vi "WHD_VEten_0.1.3.WS_BIDIR_SAI_opt.vi"() -> ()   [LabVIEW 2015]
uses:
  <vilib>/NI_Real-Time Target Support.lvlib
  <vilib>/rvi/interface/nirviReadWriteControl/nirviReadWriteControl.xnode
  <vilib>/rvi/interface/nirviMethod/nirviMethod.xnode
  <vilib>/rvi/interface/nirviOpenFPGA/nirviOpenFPGA.xnode
  <vilib>/rvi/interface/nirviCloseFPGA/nirviCloseFPGA.xnode
  <vilib>/userdefined/High Color/nirio_resource_hc.ctl
  <vilib>/rvi/errors/niLvFpgaMergeErrorWithErrorCode.vi
  <vilib>/Utility/file.llb/Write Delimited Spreadsheet (string).vi
  <vilib>/RTwatchdog.llb/Watchdog expiration actions.ctl
  AURA_Wheel/Json2Labv.lvlib
  AURA_Wheel/AuraWheelAPI/AuraWheel.lvlib
  <vilib>/rvi/errors/niLvFpgaAdjustHostInterfaceError.vi
  NiFpgaLv.dll
  <vilib>/Utility/error.llb/Error Cluster From Error Code.vi
  <vilib>/LabVIEW Targets/FPGA/cRIO/shared/nicrio_ModuleControls/nicrio_cRIO-9234_DataRatesRing2.ctl
  <vilib>/FPGAPlugInAG/cRIO-9031/niLvFpga_Run_cRIO-9031.vi
  <vilib>/FPGAPlugInAG/cRIO-9031/niLvFpga_Reset_cRIO-9031.vi
  FPGA Bitfiles/W&RDArabia_FPGATarget_FPGA8a2wsBIdirec_yJvL9yuTbZw.lvbitx
  <vilib>/Utility/config.llb/NI_LVConfig.lvlib
  <vilib>/Utility/config.llb/Write Key (Double).vi
  <vilib>/platform/TimedLoop/XDataNode/XDataNode.xnode
  <vilib>/Platform/TimedLoop/XDataNode/nitl_modes.ctl
  <vilib>/Platform/TimedLoop/XDataNode/XDNodeRunTimeDep.lvlib
  <vilib>/Platform/TimedLoop/XDataNode/wakeup.ctl
  <vilib>/Platform/TimedLoop/XDataNode/timing_clust.ctl
  <vilib>/FPGAPlugInAG/cRIO-9031/niLvFpga_Open_cRIO-9031.vi
  <vilib>/FPGAPlugInAG/cRIO-9031/niLvFpga_ConfigureFifo_cRIO-9031.vi
  <vilib>/FPGAPlugInAG/cRIO-9031/niLvFpga_StartFifo_cRIO-9031.vi
  <vilib>/FPGAPlugInAG/cRIO-9031/niLvFpga_ReadFifo_cRIO-9031.vi
  <vilib>/FPGAPlugInAG/cRIO-9031/niLvFpga_StopFifo_cRIO-9031.vi
  <vilib>/FPGAPlugInAG/cRIO-9031/niLvFpga_Close_cRIO-9031.vi
panel:
  in  "Developer commad":string
  out "Save calibration":bool
  out "calibration log":path
  out "Pattern amplitude (g)":dbl=1.02
  out "Pattern frequency (Hz)":dbl=159.2
  out "Folder":path
  out "Report":string
  out "path calib":path
  out "AURA wheel test":bool
  out "LOG.txt":path
  out "Report_AURA":string
  out "RFID_Error":errorcluster
  out "error FPGA":errorcluster
  out "error AURA":errorcluster
  out "error manipulacion archivos":errorcluster
  out "Response headers":string
  out "Max RMS Ruedas":dbl[][](array[numeric])
  out "TAGs LR6":string[](array[string])
  out "TAGs HEX":string[](array[string])
  out "Parar":bool
  out "result":bool
  out "TAGs":string[](array[string])
  out "Temperatura (ºC)":dbl
  out "V (m/s)":dbl
  out "Digital?":bool=TRUE
  out "Watchdog config":T1={"reset system"=FALSE, "restart LabVIEW Runtime"=FALSE, "occurrence"=FALSE, "trigger protocol"=enum."active high", "trigger line"=enum."none", "disable watchdog on VI exit"=TRUE}
  out "Tiempo de adquisicion":dbl=10.0
  out "Adquirir":bool
  out "Nº Ruedas 1":i32
  out "NºRuedas 2":i32
  out "Disco Duro Disponible (bytes)":i64
  out "Buffer Overflow":bool
  out "Buffer Underflow":bool
  out "Archivo\nvalido?":bool
  out "Número de ejes detectados":i32
  out "Ejes_convoy":i32
  out "Tiempo de paso (s)":dbl
  out "created path":path
  out "Nombre de archivo":path[](array[path])
  out "LR6 IP address":string="192.168.106.94"
  out "Port LR6":u16=2001
  out "T fuera rango":bool
  out "Frecuencia de muestreo (Hz)":dbl=25600.0
  out "Escaneos de la FIFO por canal":u32=5000
  out "Tiempo extra al detector de paso (s)":dbl=1.0
  out "dt RMS":dbl=256.0
  out "Frecuencia de muestreo y módulo CRIO":T2=2 items=["51.200 kS/s (NI 9234)"=1, "25.600 kS/s (NI 9234)"=2, "17.067 kS/s (NI 9234)"=3, "12.800 kS/s (NI 9234)"=4, "10.240 kS/s (NI 9234)"=5, "8.533 kS/s (NI 9234)"=6, "7.314 kS/s (NI 9234)"=7, "6.400 kS/s (NI 9234)"=8, "5.689 kS/s (NI 9234)"=9, "5.120 kS/s (NI 9234)"=10, "4.654 kS/s (NI 9234)"=11, "4.267 kS/s (NI 9234)"=12, "3.938 kS/s (NI 9234)"=13, "3.657 kS/s (NI 9234)"=14, "3.413 kS/s (NI 9234)"=15, "3.200 kS/s (NI 9234)"=16, "3.012 kS/s (NI 9234)"=17, "2.845 kS/s (NI 9234)"=18, "2.695 kS/s (NI 9234)"=19, "2.560 kS/s (NI 9234)"=20, "2.438 kS/s (NI 9234)"=21, "2.328 kS/s (NI 9234)"=22, "2.226 kS/s (NI 9234)"=23, "2.133 kS/s (NI 9234)"=24, "2.048 kS/s (NI 9234)"=25, "1.969 kS/s (NI 9234)"=26, "1.896 kS/s (NI 9234)"=27, "1.829 kS/s (NI 9234)"=28, "1.765 kS/s (NI 9234)"=29, "1.707 kS/s (NI 9234)"=30, "1.652 kS/s (NI 9234)"=31]
  out "Puerto RFID":u16=2189
  out "IP RFID":string="192.168.106.99"
  out "Offset_rueda WS 2":fxp<+/-,24,-4>=0.004999998956918716 format="%.27g"
  out "Count(mSec)":u32=2
  out "RFID NEM on?":bool
  out "RFID LR6 on?":bool
  out "Canal cero WS1?":bool
  out "Canal cero WS2":bool
  out "Inicio pasada 2":timestamp
  in  "Calibration":bool
  out "Direccion 0?":bool
  out "Boton Adquirir?":bool
  out "RuedaDetectada2?":bool=TRUE
  out "RuedaDetectada1?":bool=TRUE
  out "Timeout ruedas":dbl
  out "Borrar archivos\nadquisicion con error":bool
  out "Able watchdog?":bool
  out "Reset watchdog?":bool
  out "Leer config RFID NEM":bool
  out "bytes to read":i32
  out "DeviceAddress":u8
  out "timeout ms (60000)":i32
  out "Max archivos":u32=2
  out "Bytes libre despues de borrar":u32=2
  out "Bytes min libre":u32=2
  out "Nº de acelerómetros":i32
  out "Nº inductivos":i32
  out "Offset_rueda WS 1":fxp<+/-,24,-4>=0.004999998956918716 format="%.27g"
  out "TAGs_AURAwheel":string[][](array[string])
  out "Plataformas?":bool
  out "Nº Ejes":i32[](array[numeric])
  out "Nº UTs":i32
  out "it-read-LR6":i32[](array[numeric])
  out "it-LR6":i32
  out "RFID_LR6_Error":errorcluster
  out "Series_flota":string[](array[string])
  out "Tabla_flota":string[][](array[string])
  out "Puntos medios de las ventanas":dbl[][](array[numeric])
  out "configuration file path":path=path "c:/Parametros.cfg"
  out "IP synchr":string
  out "data":cluster{"status":string}
  out "confRFID":path=path "c:/RFID/TAGS.csv"
  out "TAGS leidos":path=path "c:/RFID/TAGS.csv"
  out "Use Aura?":bool
  out "Parametros AuraWheel":string[](array[string])
  out "Parámetros acelerómetros":dbl[](array[numeric])
  out "Fin":bool
  out "Contador":i32=1
  out "Path LOG":path=path "c:/TEST"
  out "Fallo fotocelula":bool
  out "Path_Borrar":path=path "c:/Trenes"
  out "Longitud de la unidad":dbl
  out "Aviso no detección":string
  out "Time to Acquire Block (ms)":i32
  out "Distancia de acelerómetros":dbl[](array[numeric])
  out "Block Size":u32
  out "Distancias generales":dbl[](array[numeric])
  out "Reset del controlador":bool
  out "Parar la aplicación":bool
  out "date/time string":string
  out "Timeout ruedas":bool
  out "Tiempo":dbl
  out "Inicio pasada":timestamp
  out "Ultimo TEST":timestamp
  out "Fuente":bool=TRUE
  out "RFID_ID":refnum<k5>
  out "DC OK":string
  out "Aviso temperatura":string
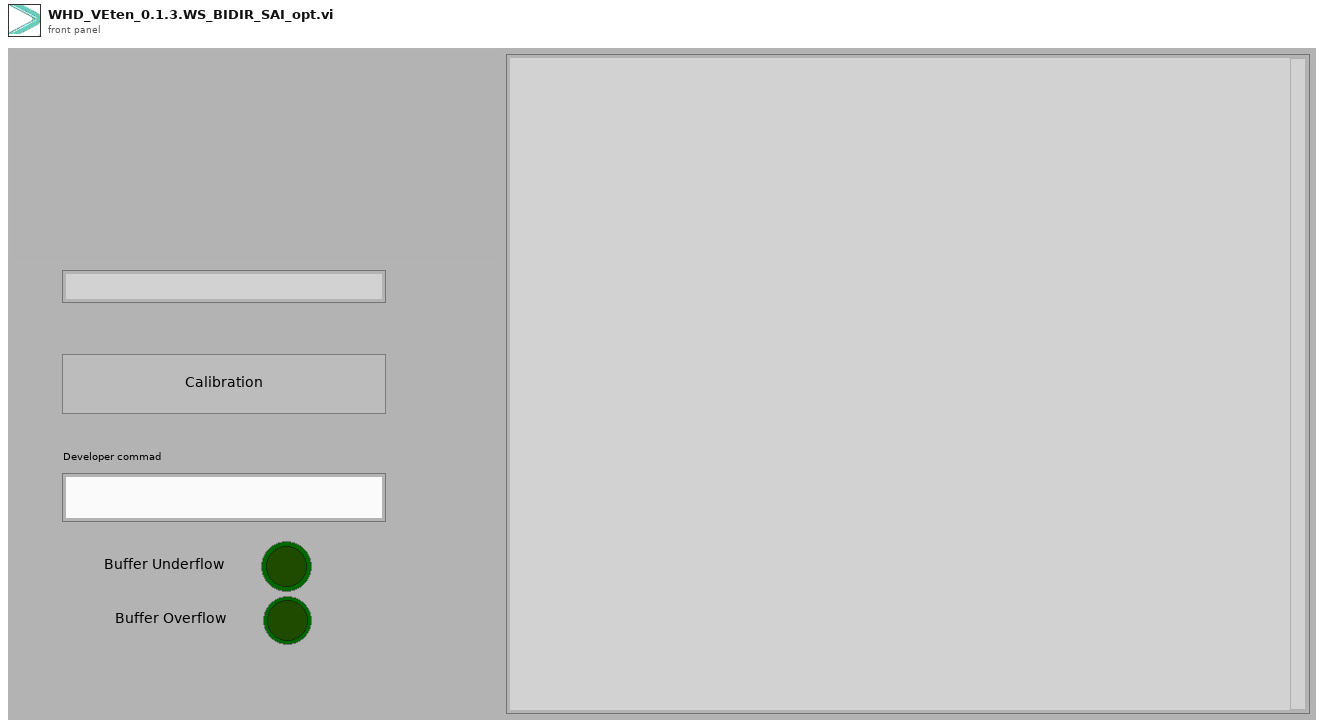
[diagram p1: front panel]
types:
  T1 = typedef "Watchdog expiration actions.ctl" = cluster{"reset system":bool, "restart LabVIEW Runtime":bool, "occurrence":bool, "trigger protocol":enum16{"active high", "active low", "open collector"}, "trigger line":enum16{"none", "line 0", "line 1", "line 2", "line 3", "line 4", "line 5", "line 6", "line 7", "SMB line 0"}, "disable watchdog on VI exit":bool}
  T2 = typedef "nicrio_cRIO-9234_DataRatesRing2.ctl" = u8
  T3 = typedef "nirio_resource_hc.ctl" = tag
  T4 = enum16{"Standard", "Buffered", "CRLF", "Immediate"}
  T5 = enum16{"open", "replace", "create", "open or create", "replace or create", "replace or create with confirmation"}
  T6 = enum16{"big-endian, network order", "native, host order", "little-endian"}
  T7 = typedef "XDNodeRunTimeDep.lvlib/timing_clust.ctl" = cluster{"Expected End [f-1]":u64, "Actual End [f-1]":u64, "Finished Late? [f-1]":bool, "Expected End [i-1]":u64, "Actual End [i-1]":u64, "Finished Late? [i-1]":bool, "Expected Start [i]":u64, "Actual Start [i]":u64, "Expected Start [f]":u64, "Actual Start [f]":u64, "Source Name":string, "Structure Name":string, "Period":i64, "Deadline":i64, "Offset":i64, "Start":i64, "Priority":i32, "Timeout":i32, "Mode":T8, "Wakeup Reason":T9, "Error":errorcluster, "Source Type":string, "Secondary Source Type":string, "Global End Time":u64, "Global Start Time":u64, "Frame Duration":u64, "Iteration Duration":u64, "Assigned CPU":i32, "I/O Scan Engine Mode":u32}
  T8 = typedef "XDNodeRunTimeDep.lvlib/nitl_modes.ctl" = enum32{"No Change", "Process missed periods, maintain original phase", "Discard missed periods, maintain original phase", "Process missed periods, ignore original phase", "Discard missed periods, ignore original phase"}
  T9 = typedef "XDNodeRunTimeDep.lvlib/wakeup.ctl" = enum32{"Normal", "Aborted", "Asynchronous wakeup", "Timing source error", "Timed loop error", "Timeout"}
  T10 = cluster{"error IO":errorcluster, bool[], u32[], string[], dbl[]}
  T11 = cluster{"error out":errorcluster, dbl[], "TAGs":string[], "Direccion 0?":bool}
  T12 = cluster{"g_ts":dbl, "p_sp":dbl, "p_tp":dbl, "p_tg":cluster{"tg_n":dbl, "tg_t":string}[], "p_ax":cluster{"ax_n":dbl, "ax_sp":dbl, "ax_wh":cluster{"wh_p":dbl, "wh_a1":dbl, "wh_a2":dbl, "wh_a3":dbl, "wh_a4":dbl}[]}[]}
  T13 = cluster{"Frecuencia de muestreo y módulo CRIO":T2, "Count(mSec)":u32, "Frecuencia de muestreo (Hz)":dbl, "Escaneos de la FIFO por canal":u32, "Nº inductivos":i32, "Nº de acelerómetros":i32}
  T14 = typedef "NI_LVConfig.lvlib/Config Data RefNum.ctl" = refnum<k1>
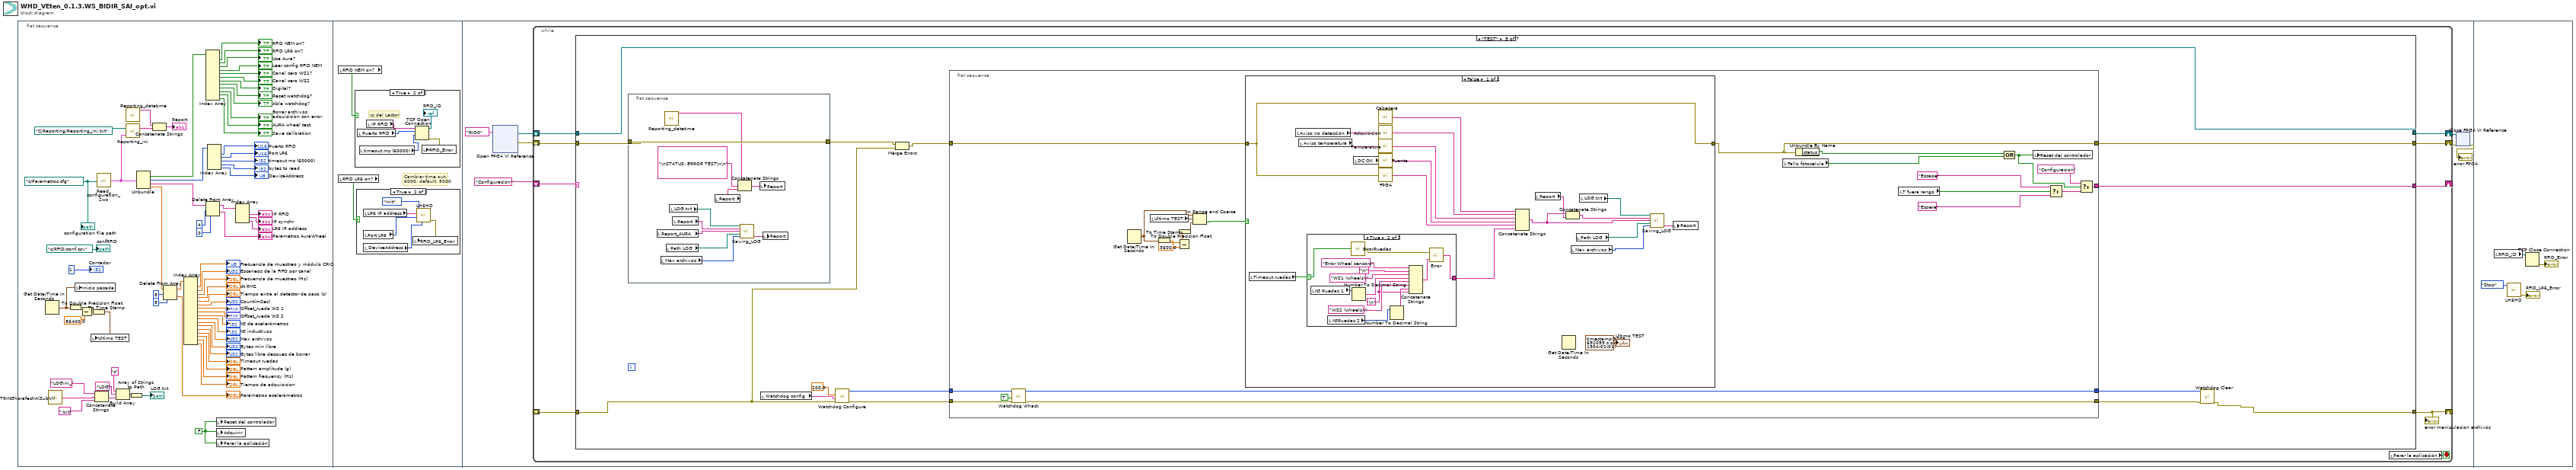
[diagram p0: block diagram]
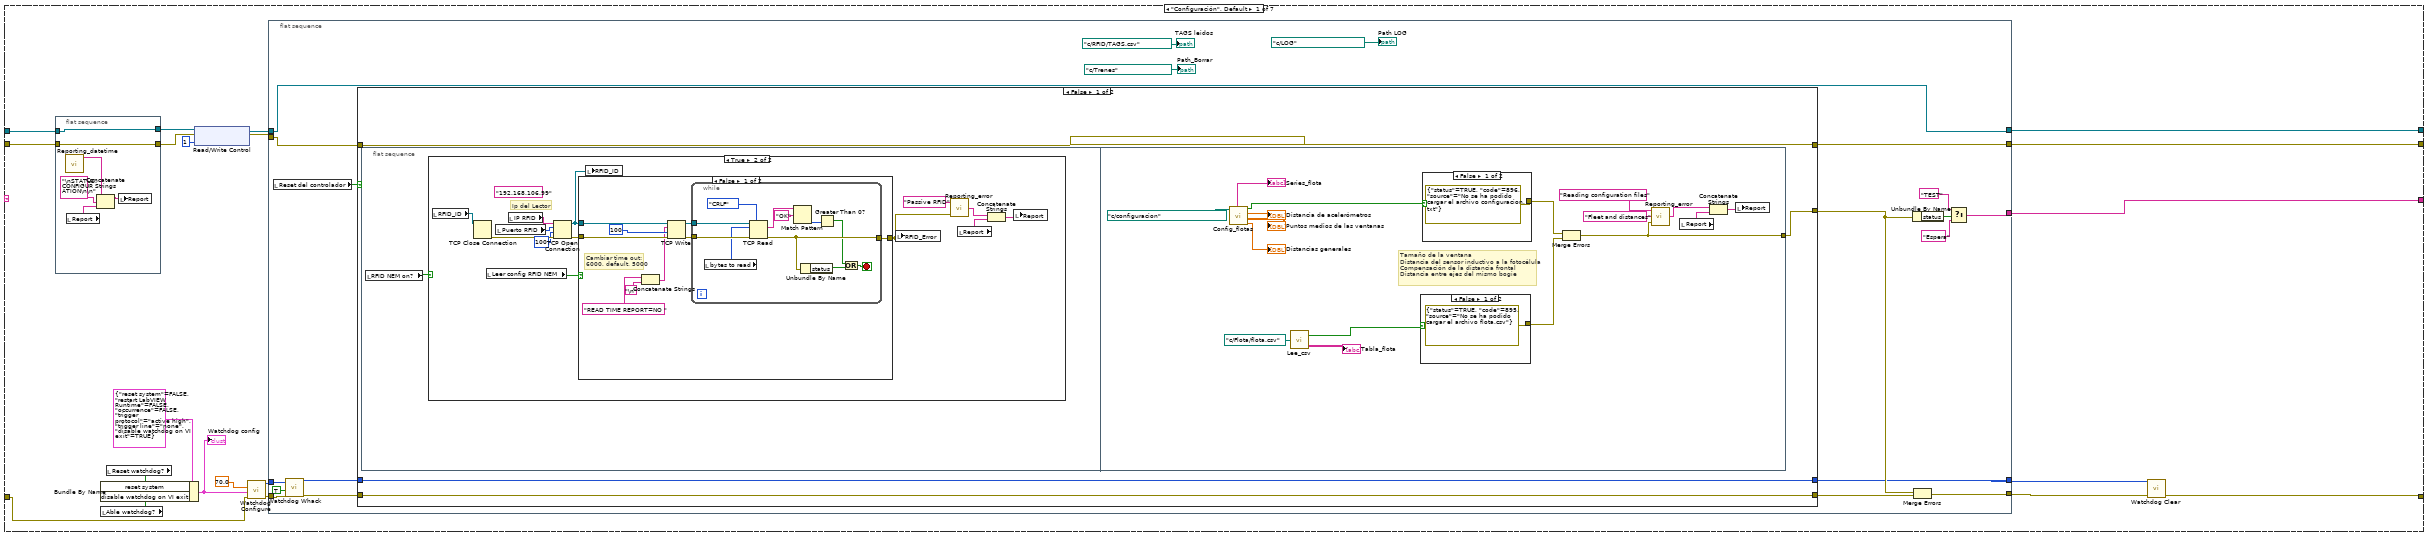
[diagram p4: hidden frame]
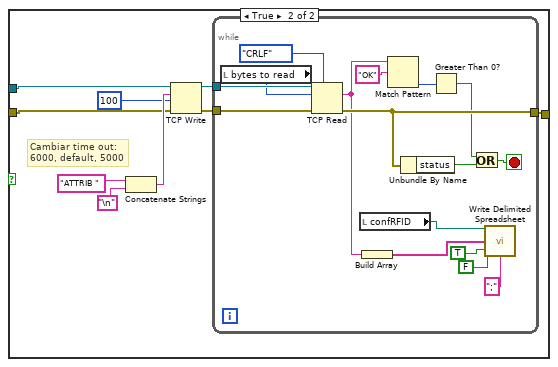
[diagram p6: hidden frame]
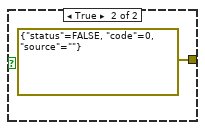
[diagram p7: hidden frame]
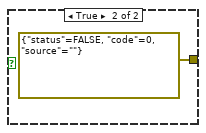
[diagram p8: hidden frame]
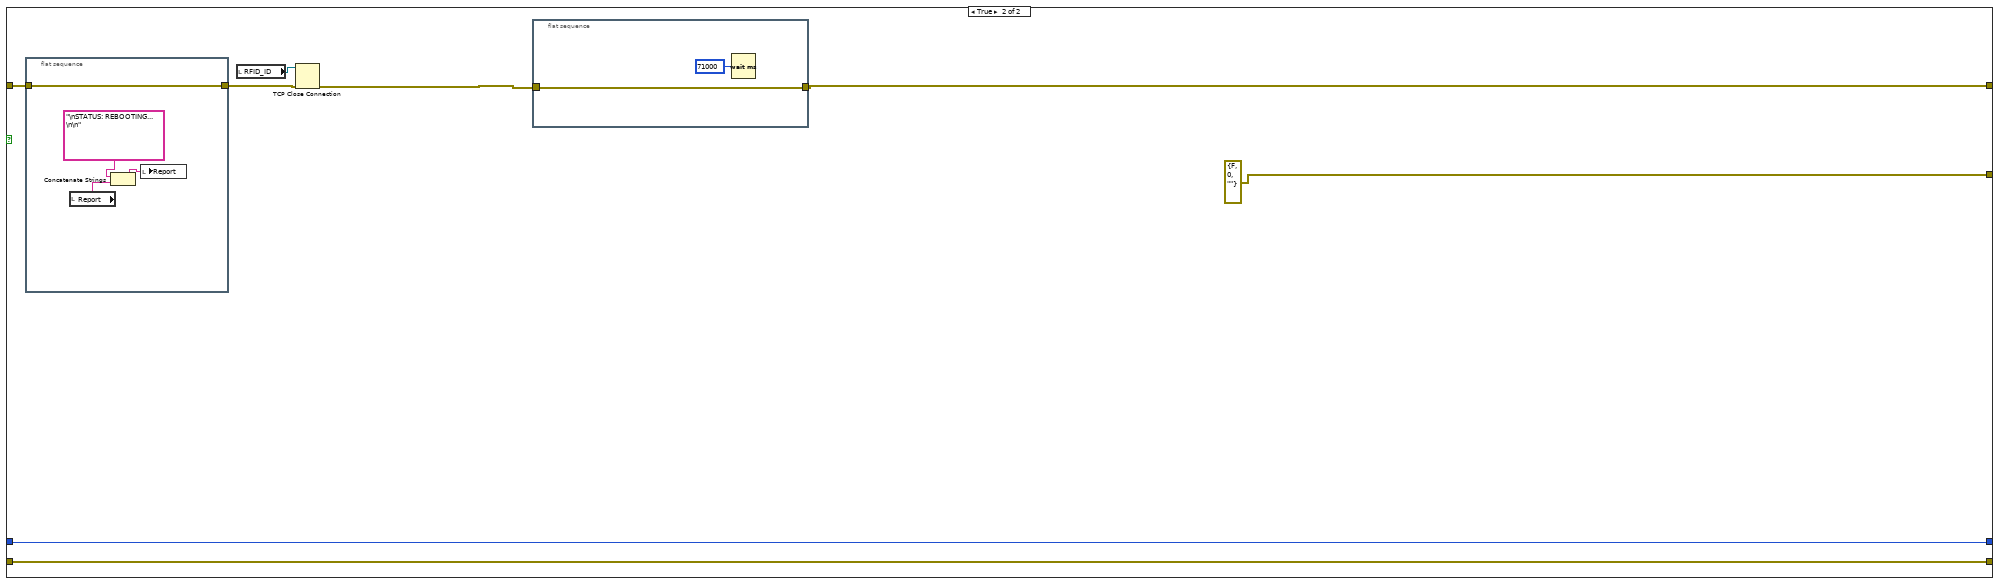
[diagram p9: hidden frame]
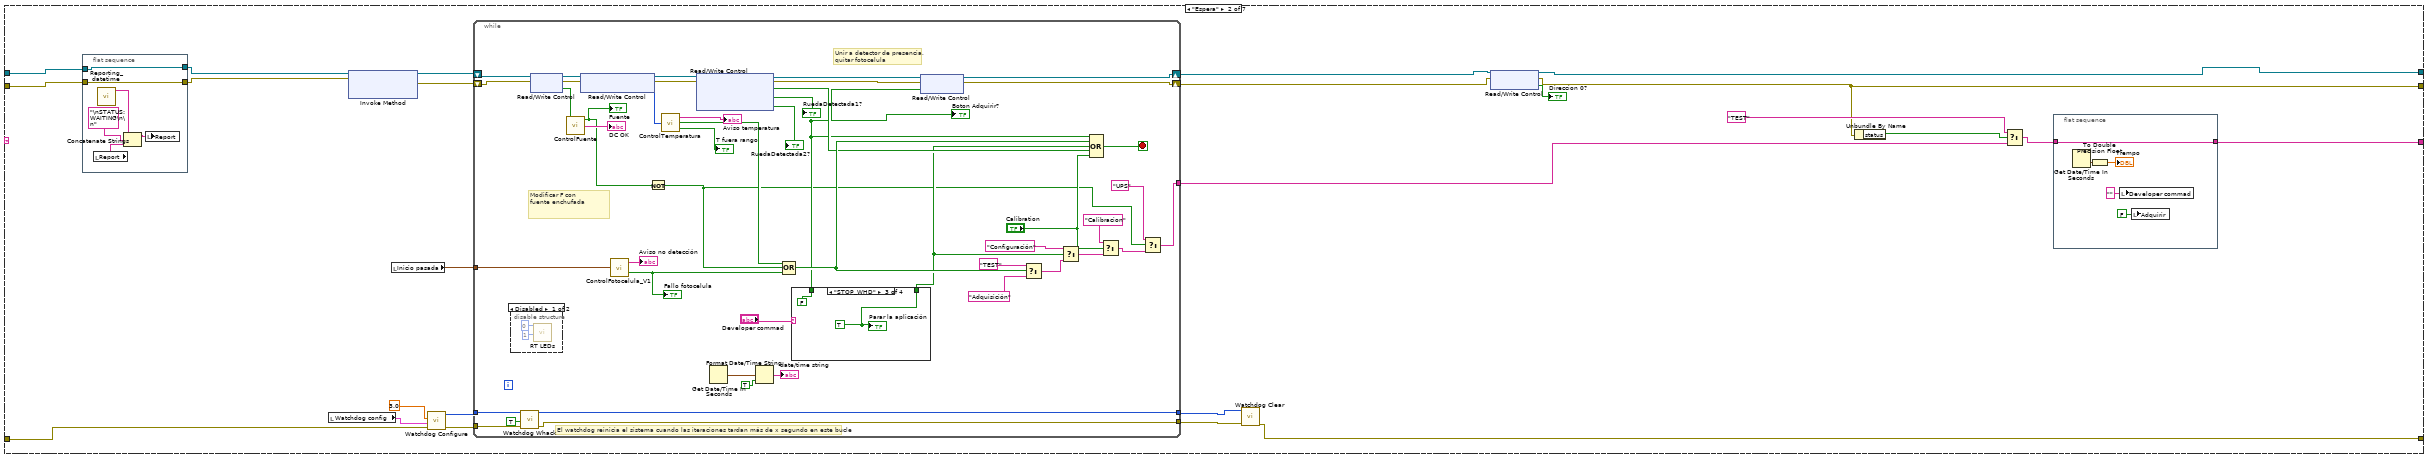
[diagram p10: hidden frame]
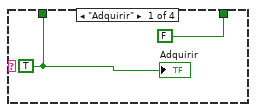
[diagram p11: hidden frame]
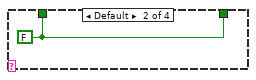
[diagram p12: hidden frame]
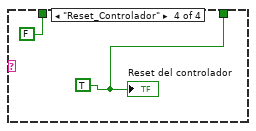
[diagram p13: hidden frame]
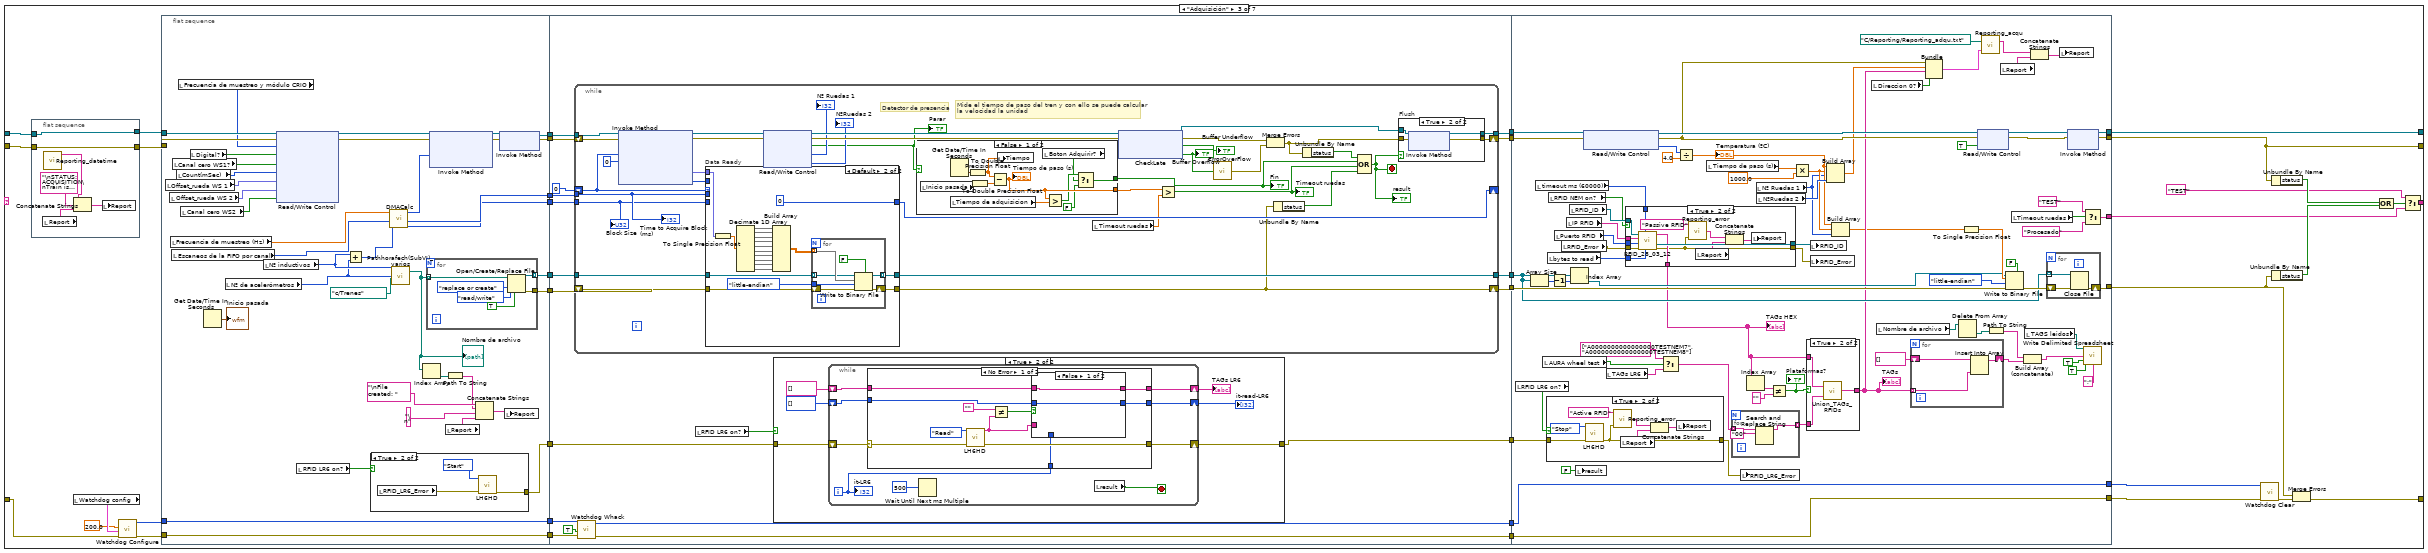
[diagram p15: hidden frame]
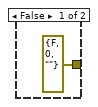
[diagram p16: hidden frame]
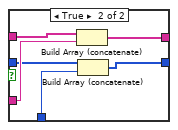
[diagram p18: hidden frame]
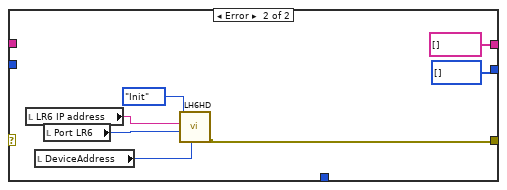
[diagram p19: hidden frame]
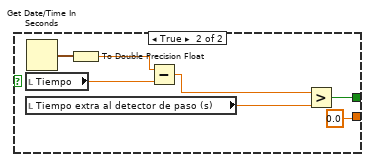
[diagram p20: hidden frame]
diagram:
  n1 = flat-sequence {
    frame #0 {
      w1 = FALSE ("Reset del controlador")
      w63 = path "c:/Parametros.cfg" ("configuration file path")
      n2 = Get Date/Time In Seconds() -> (seconds since 1Jan1904=w68:timestamp)
      n3 = call "STRINGhorafechA(SubVI).vi"() -> ("STRINGhora_fecha"=w12:string)
      n4 = To Double Precision Float(number=w68) -> (double precision float=w70:dbl)
      n5 = local write "Inicio pasada"(w68) -> ()
      n6 = Subtract(x=w70, y=86400.0) -> (x-y=w69:dbl)
      n7 = To Time Stamp(1:w69) -> (0:w67:timestamp)
      n8 = local write "Ultimo TEST"(w67) -> ()
      n9 = Concatenate Strings("LOGini_" ("string"), w12, ".txt" ("string")) -> (w14:string)
      n10 = call "Read_configuration_2ws.vi"("configuration file path"=w63) -> ("output cluster"=w18:T10)
      n11 = Build Array("c", "LOG" ("element"), w14) -> (w11:string[])
      n12 = call "Reporting_ini.vi"("Configuration cluster"=w18, "address repoting"=path "C:/Reporting/Reporting_ini.txt" ("file (use dialog)")) -> ("Reporting"=w17:string)  [unwired: 1 in]
      n13 = call "Reporting_datetime.vi"() -> ("String"=w15:string)  [unwired: 11 in]
      n14 = Array of Strings to Path(0:w11) -> (2:→"LOG.txt":path)  [unwired: 1 out]
      n15 = Unbundle(w18) -> (w66:bool[], w65:u32[], w58:string[], w62:dbl[])  [unwired: 1 out]
      n16 = Concatenate Strings(w15, w17) -> (→"Report":string)
      n17 = Delete From Array(array=w62, length=8, index=8) -> (deleted portion=→"Parámetros acelerómetros":dbl[], array with subset deleted=w61:dbl[])
      n18 = Index Array(array=w61) -> (element #1=→"Frecuencia de muestreo y módulo CRIO":dbl, element #2=→"Escaneos de la FIFO por canal":dbl, element #3=→"Frecuencia de muestreo (Hz)":dbl, element #4=→"dt RMS":dbl, element #5=→"Tiempo extra al detector de paso (s)":dbl, element #6=→"Count(mSec)":dbl, element #7=→"Offset_rueda WS 1":dbl, element #8=→"Offset_rueda WS 2":dbl, element #9=→"Nº de acelerómetros":dbl, element #10=→"Nº inductivos":dbl, element #11=→"Max archivos":dbl, element #12=→"Bytes min libre":dbl, element #13=→"Bytes libre despues de borrar":dbl, element #14=→"Timeout ruedas":dbl, element #15=→"Pattern amplitude (g)":dbl, element #16=→"Pattern frequency (Hz)":dbl, element #17=→"Tiempo de adquisicion":dbl)  [unwired: 17 in]
      n19 = Index Array(array=w66) -> (element #1=→"RFID NEM on?":bool, element #2=→"RFID LR6 on?":bool, element #3=→"Use Aura?":bool, element #4=→"Leer config RFID NEM":bool, element #5=→"Canal cero WS1?":bool, element #6=→"Canal cero WS2":bool, element #7=→"Digital?":bool, element #8=→"Reset watchdog?":bool, element #9=→"Able watchdog?":bool, element #10=→"Borrar archivos\nadquisicion con error":bool, element #11=→"AURA wheel test":bool, element #12=→"Save calibration":bool)  [unwired: 12 in]
      n20 = Delete From Array(array=w58, length=4, index=0) -> (deleted portion=→"Parametros AuraWheel":string[], array with subset deleted=w57:string[])
      n21 = Index Array(array=w65) -> (element #1=→"Puerto RFID":u32, element #2=→"Port LR6":u32, element #3=→"timeout ms (60000)":u32, element #4=→"bytes to read":u32, element #5=→"DeviceAddress":u32)  [unwired: 5 in]
      n22 = local write "Reset del controlador"(w1) -> ()
      n23 = local write "Adquirir"(w1) -> ()
      n24 = local write "Parar la aplicación"(w1) -> ()
      n25 = Index Array(array=w57) -> (element #1=→"IP RFID":string, element #2=→"IP synchr":string, element #3=→"LR6 IP address":string)  [unwired: 3 in]
      "Contador" <- 1
      "confRFID" <- path "c:/RFID/conf.csv" ("file path (use dialog)")
      "configuration file path" <- w63
    }
    frame #1 {
      # "Cambiar time out:\n6000, default, 5000"
      n26 = local read "RFID NEM on?"() -> (w73:bool)
      n27 = local read "RFID LR6 on?"() -> (w72:bool)
      n28 = case shown="True" w73 {
        frame False {
        }
        frame True {
          # "Ip del Lector"
          n29 = local read "Puerto RFID"() -> (w81:u16)
          n30 = local read "timeout ms (60000)"() -> (w79:i32)
          n31 = local read "IP RFID"() -> (w82:string)
          n32 = TCP Open Connection(address=w82, remote port or service name=w81, timeout ms (60000)=w79) -> (connection ID=→"RFID_ID":refnum<k5>, error out=w80:errorcluster)  [unwired: 1 in, 1 out]
          n33 = local write "RFID_Error"(w80) -> ()
        }
      }
      n34 = case shown="True" w72 {
        frame False {
        }
        frame True {
          n35 = local read "LR6 IP address"() -> (w74:string)
          n36 = local read "Port LR6"() -> (w75:u16)
          n37 = local read "DeviceAddress"() -> (w76:u8)
          n38 = call "LH6HD.vi"("DeviceAddress"=w76, "Reader Port"=w75, "IP Address"=w74, "Action"=enum16{"Init", "Start", "Read", "Stop", "Exit"}."Init") -> ("error out"=w78:errorcluster)  [unwired: 6 in, 1 out]
          n39 = local write "RFID_LR6_Error"(w78) -> ()
        }
      }
    }
    frame #2 {
      n40 = xnode "Open FPGA VI Reference"("resource name"=T3 "RIO0") -> ("FPGA VI Reference Out"=w90:refnum<k20>, "error out"=w89:errorcluster)  [unwired: 1 in]
      n41 = while {
        shift-right: [w91] -> _
        shift-left: "Configuración" -> [w99]
        shift-right: [w93] -> w86
        shift-left: w90 -> [w98]
        shift-right: [w92] -> w85
        shift-left: w89 -> [w97]
        shift-right: [w96] -> _
        shift-left: _ -> [w95]
        stop <- w94 stop-if-true
        n42 = case shown="\"TEST\"" w99 {
          tunnel: [w109 w262 w354 w711 w959 "Espera" "Espera" ("t")] -> w91
          tunnel: [w119 w250 w368 w700 w958 w1038 w1229] -> w93
          tunnel: [w120 w249 w369 w698 w957 w1037 w1228] -> w92
          tunnel: w98 -> [w103 w248 w340 w701 w958 w1043 w1232]
          tunnel: w97 -> [w102 w247 w339 w699 w950 w1042 w1231]
          tunnel: [w116 w256 w366 w696 w949 _ _] -> w96
          tunnel: w95 -> [w108 w261 w350 w710 w946 _ _]
          frame "Configuración", Default {
            n43 = flat-sequence {
              tunnel: w103 -> [w126]
              tunnel: w102 -> [w125]
              tunnel: [w126] -> w101
              tunnel: [w125] -> w100
              frame #0 {
                n44 = call "Reporting_datetime.vi"() -> ("String"=w121:string)  [unwired: 11 in]
                n45 = local read "Report"() -> (w122:string)
                n46 = Concatenate Strings(w121, "\nSTATUS: CONFIGURATION\n\n", w122) -> (w124:string)
                n47 = local write "Report"(w124) -> ()
              }
            }
            n48 = local read "Able watchdog?"() -> (w113:bool)
            n49 = local read "Reset watchdog?"() -> (w114:bool)
            n50 = Bundle By Name(cluster=T1 {"reset system"=FALSE, "restart LabVIEW Runtime"=FALSE, "occurrence"=FALSE, "trigger protocol"=enum."active high", "trigger line"=enum."none", "disable watchdog on VI exit"=TRUE} ("expiration actions"), "reset system"=w114, "disable watchdog on VI exit"=w113) -> (w107:T1)
            "Watchdog config" <- w107
            n51 = xnode "Read/Write Control"("FPGA VI Reference In"=w101, "error in"=w100, "Cycles to Filter"=u16 1) -> ("FPGA VI Reference Out"=w112:refnum<k20>, "error out"=w111:errorcluster)
            n52 = call <vilib>:"Watchdog Configure.vi"("error in (no error)"=w108, "expiration actions"=w107, "timeout (1 sec)"=70.0) -> ("error out"=w104:errorcluster, "watchdogID"=w105:u64)  [unwired: 1 in, 2 out]
            n53 = flat-sequence {
              tunnel: [w137] -> w120
              tunnel: [w145] -> w109
              tunnel: w112 -> [w138]
              tunnel: [w138] -> w119
              tunnel: [w140] -> w117
              tunnel: w111 -> [w135]
              tunnel: [w132] -> w118
              tunnel: w105 -> [w128]
              tunnel: w104 -> [w127]
              frame #0 {
                n54 = local read "Reset del controlador"() -> (w134:bool)
                n55 = call <vilib>:"Watchdog Whack.vi"("error in (no error)"=w127, "reset watchdog after expire? (F)"=TRUE, "watchdogID in"=w128) -> ("error out"=w130:errorcluster, "watchdogID out"=w131:u64)  [unwired: 2 in, 1 out]
                n56 = case shown="False" w134 {
                  tunnel: w135 -> [w150 w233]
                  tunnel: [w150 w236] -> w137
                  tunnel: [w147 errorcluster {"status"=FALSE, "code"=0, "source"=""} ("error IO")] -> w136
                  tunnel: [w149 w235] -> w132
                  tunnel: w131 -> [w149 w235]
                  tunnel: w130 -> [w148 w234]
                  tunnel: [w148 w234] -> w129
                  frame False {
                    n57 = flat-sequence {
                      tunnel: [w210] -> w147
                      frame #0 {
                        n58 = local read "RFID NEM on?"() -> (w151:bool)
                        n59 = case shown="True" w151 {
                          frame False {
                          }
                          frame True {
                            (unwired) "192.168.106.99" ("address")
                            # "Ip del Lector"
                            n60 = local read "RFID_ID"() -> (w163:refnum<k5>)
                            n61 = TCP Close Connection(connection ID=w163) -> (error out=w164:errorcluster)  [unwired: 2 in, 1 out]
                            n62 = local read "Leer config RFID NEM"() -> (w157:bool)
                            n63 = local read "Puerto RFID"() -> (w161:u16)
                            n64 = local read "IP RFID"() -> (w160:string)
                            n65 = TCP Open Connection(address=w160, remote port or service name=w161, timeout ms (60000)=100, error in (no error)=w164) -> (connection ID=w162:refnum<k5>, error out=w158:errorcluster)  [unwired: 1 out]
                            n66 = case shown="False" w157 {
                              tunnel: w162 -> [w173 w187]
                              tunnel: [w171 w185] -> w156
                              tunnel: w158 -> [w168 w186]
                              frame False {
                                # "Cambiar time out:\n6000, default, 5000"
                                n67 = Concatenate Strings("READ TIME REPORT=NO " ("data in"), "\n") -> (w165:string)
                                n68 = TCP Write(connection ID=w173, data in=w165, error in (no error)=w168, 9:100 ("timeout ms (25000)")) -> (connection ID out=w169:refnum<k5>, error out=w170:errorcluster)  [unwired: 1 out]
                                n69 = while {
                                tunnel: w170 -> [w183]
                                tunnel: w169 -> [w182]
                                tunnel: [w181] -> w171
                                stop <- w178 stop-if-true
                                n70 = local read "bytes to read"() -> (w174:i32)
                                n71 = TCP Read(connection ID=w182, bytes to read=w174, error in (no error)=w183, 7:T4."CRLF" ("mode (standard)")) -> (data out=w176:string, error out=w181:errorcluster)  [unwired: 1 in, 1 out]
                                n72 = Match Pattern(string=w176, regular expression="OK") -> (offset past match=w179:i32)  [unwired: 4 out]
                                n73 = Unbundle By Name(w181) -> ("status"=w177:bool)
                                n74 = Greater Than 0?(x=w179) -> (x > 0?=w175:bool)
                                n75 = Or(x=w175, y=w177) -> (x .or. y?=w178:bool)
                                }
                              }
                              frame True {
                                # "Cambiar time out:\n6000, default, 5000"
                                n76 = Concatenate Strings("ATTRIB " ("data in"), "\n") -> (w193:string)
                                n77 = TCP Write(connection ID=w187, data in=w193, error in (no error)=w186, 9:100 ("timeout ms (25000)")) -> (connection ID out=w190:refnum<k5>, error out=w189:errorcluster)  [unwired: 1 out]
                                n78 = while {
                                tunnel: w189 -> [w208]
                                tunnel: w190 -> [w207]
                                tunnel: [w206] -> w185
                                stop <- w203 stop-if-true
                                n79 = local read "bytes to read"() -> (w194:i32)
                                n80 = TCP Read(connection ID=w207, bytes to read=w194, error in (no error)=w208, 7:T4."CRLF" ("mode (standard)")) -> (data out=w197:string, error out=w206:errorcluster)  [unwired: 1 in, 1 out]
                                n81 = local read "confRFID"() -> (w196:path)
                                n82 = Build Array(w197) -> (w195:string[])
                                n83 = Match Pattern(string=w197, regular expression="OK") -> (offset past match=w204:i32)  [unwired: 4 out]
                                n84 = Unbundle By Name(w206) -> ("status"=w202:bool)
                                n85 = Greater Than 0?(x=w204) -> (x > 0?=w201:bool)
                                n86 = Or(x=w201, y=w202) -> (x .or. y?=w203:bool)
                                n87 = call-poly <vilib>:"Write Delimited Spreadsheet.vi"("file path (dialog if empty)"=w196, "1D data"=w195, "append to file? (new file:F)"=FALSE ("transpose? (no:F)"), "transpose? (no:F)"=TRUE ("append to file? (new file:F)"), "delimiter (\\t)"=";" ("delimiter (\\t)")) -> ()  [unwired: 9 in, 2 out]
                                }
                              }
                            }
                            n88 = local write "RFID_ID"(w162) -> ()
                            n89 = local write "RFID_Error"(w156) -> ()
                            n90 = call "Reporting_error.vi"("error out 2"=w156, "Concept"="Passive RFID") -> ("Reporting"=w153:string)  [unwired: 1 in]
                            n91 = local read "Report"() -> (w154:string)
                            n92 = Concatenate Strings(w153, w154) -> (w152:string)
                            n93 = local write "Report"(w152) -> ()
                          }
                        }
                      }
                      frame #1 {
                        # "Tamaño de la ventana\nDistancia del sensor inductivo a la fotocélula\nCompensación de la distancia frontal\nDistancia entre ejes del mismo bogie"
                        n94 = call "Config_flotas.vi"("file path (dialog if empty)"=path "c:/configuracion") -> ("Distancias generales"=→"Distancias generales":dbl[], "Puntos medios de las ventanas"=→"Puntos medios de las ventanas":dbl[][], "Distancia de acelerómetros"=→"Distancia de acelerómetros":dbl[], "Distacias y medidas de dispositivos"=w223:bool, "Series_flota"=→"Series_flota":string[])  [unwired: 3 in]
                        n95 = call "Lee_csv.vi"("Path"=path "c:/Flota/flota.csv") -> ("Tabla_flota"=→"Tabla_flota":string[][], "Lectura_OK?"=w220:bool)
                        n96 = case shown="False" w220 {
                          tunnel: [errorcluster {"status"=TRUE, "code"=895, "source"="No se ha podido cargar el archivo flota.csv"} ("error out") errorcluster {"status"=FALSE, "code"=0, "source"=""} ("error out")] -> w224
                          frame False {
                          }
                          frame True {
                          }
                        }
                        n97 = case shown="False" w223 {
                          tunnel: [errorcluster {"status"=TRUE, "code"=896, "source"="No se ha podido cargar el archivo configuracion.txt"} ("error out") errorcluster {"status"=FALSE, "code"=0, "source"=""} ("error out")] -> w225
                          frame False {
                          }
                          frame True {
                          }
                        }
                        n98 = Merge Errors(w225, w224) -> (w210:errorcluster)
                        n99 = call "Reporting_error.vi"("error out 2"=w210, "Concept explanation"="Fleet and distances", "Concept"="Reading configuration files") -> ("Reporting"=w212:string)
                        n100 = local read "Report"() -> (w211:string)
                        n101 = Concatenate Strings(w212, w211) -> (w213:string)
                        n102 = local write "Report"(w213) -> ()
                      }
                    }
                  }
                  frame True {
                    n103 = flat-sequence {
                      tunnel: w233 -> [w242]
                      tunnel: [w242] -> w232
                      frame #0 {
                        n104 = local read "Report"() -> (w241:string)
                        n105 = Concatenate Strings("\nSTATUS: REBOOTING...\n\n", w241) -> (w239:string)
                        n106 = local write "Report"(w239) -> ()
                      }
                    }
                    n107 = local read "RFID_ID"() -> (w238:refnum<k5>)
                    n108 = TCP Close Connection(connection ID=w238, error in (no error)=w232) -> (error out=w231:errorcluster)  [unwired: 2 out]
                    n109 = flat-sequence {
                      tunnel: [w244] -> w236
                      tunnel: w231 -> [w244]
                      frame #0 {
                        n110 = Wait (ms)(milliseconds to wait=u32 71000) -> ()  [unwired: 1 out]
                      }
                    }
                  }
                }
                n111 = Unbundle By Name(w136) -> ("status"=w146:bool)
                n112 = Merge Errors(w136, w129) -> (w140:errorcluster)
                n113 = Select(t="TEST", s=w146, f="Espera") -> (s? t:f=w145:string)
                "Path_Borrar" <- path "c:/Trenes" ("file path (use dialog)")
                "Path LOG" <- path "c:/LOG" ("file path (use dialog)")
                "TAGS leidos" <- path "c:/RFID/TAGS.csv" ("file path (use dialog)")
              }
            }
            n114 = call <vilib>:"Watchdog Clear.vi"("error in (no error)"=w117, "watchdogID in"=w118) -> ("error out"=w116:errorcluster)  [unwired: 5 in]
          }
          frame "Espera" {
            n115 = flat-sequence {
              tunnel: w248 -> [w275]
              tunnel: w247 -> [w274]
              tunnel: [w275] -> w246
              tunnel: [w274] -> w245
              frame #0 {
                n116 = local read "Report"() -> (w271:string)
                n117 = call "Reporting_datetime.vi"() -> ("String"=w270:string)  [unwired: 11 in]
                n118 = Concatenate Strings(w270, "\nSTATUS: WAITING\n\n", w271) -> (w273:string)
                n119 = local write "Report"(w273) -> ()
              }
            }
            n120 = local read "Watchdog config"() -> (w255:T1)
            n121 = xnode "Invoke Method"("FPGA VI Reference In"=w246, "error in"=w245) -> ("FPGA VI Reference Out"=w265:refnum<k20>, "error out"=w264:errorcluster)  [unwired: 1 in]
            n122 = local read "Inicio pasada"() -> (w269:timestamp)
            n123 = call <vilib>:"Watchdog Configure.vi"("error in (no error)"=w261, "expiration actions"=w255, "timeout (1 sec)"=3.0) -> ("error out"=w260:errorcluster, "watchdogID"=w259:u64)  [unwired: 1 in, 2 out]
            n124 = while {
              tunnel: [w282] -> w268
              shift-right: [w299] -> w251
              shift-left: w265 -> [w307]
              shift-right: [w298] -> w252
              shift-left: w264 -> [w306]
              tunnel: w269 -> [w310]
              tunnel: w260 -> [w296]
              tunnel: w259 -> [w297]
              tunnel: [w295] -> w258
              tunnel: [w294] -> w257
              stop <- w289 stop-if-true
              # "Modificar F con\nfuente enchufada"
              # "Unir a detector de presencia,\nquitar fotocelula"
              # "El watchdog reinicia el sistema cuando las iteraciones tardan más de x segundo en este bucle"
              n125 = disable-structure shown="Disabled" {
                frame Disabled {
                  n126 = call <vilib>:"RT LEDs.vi"("State"=1, "LED Num"=0) -> ()  [unwired: 1 in, 5 out]
                }
                frame Enabled {
                }
              }
              n127 = call <vilib>:"Watchdog Whack.vi"("error in (no error)"=w296, "reset watchdog after expire? (F)"=TRUE, "watchdogID in"=w297) -> ("error out"=w294:errorcluster, "watchdogID out"=w295:u64)  [unwired: 2 in, 1 out]
              n128 = xnode "Read/Write Control"("FPGA VI Reference In"=w307, "error in"=w306) -> ("FPGA VI Reference Out"=w319:refnum<k20>, "error out"=w318:errorcluster, "DC OK"=w323:bool)
              n129 = call "ControlFuente.vi"("DC OK 3"=w323) -> ("DC OK 2"=w283:bool, "DC OK"=→"DC OK":string)  [unwired: 1 out]
              "Fuente" <- w283
              n130 = xnode "Read/Write Control"("FPGA VI Reference In"=w319, "error in"=w318) -> ("FPGA VI Reference Out"=w314:refnum<k20>, "error out"=w313:errorcluster, "Chassis Temperature"=w321:i16)
              n131 = call "ControlFotocelula_V1.vi"("Tiempo de entrada a espera"=w310) -> ("Aviso no detección"=→"Aviso no detección":string, "Boolean"=w311:bool)
              "Fallo fotocelula" <- w311
              n132 = Not(x=w283) -> (.not. x?=w281:bool)
              n133 = call "ControlTemperatura.vi"("Chassis Temperature"=w321) -> ("Aviso temperatura"=→"Aviso temperatura":string, "Boolean"=w315:bool, "T fuera rango"=→"T fuera rango":bool)
              n134 = xnode "Read/Write Control"("FPGA VI Reference In"=w314, "error in"=w313) -> ("FPGA VI Reference Out"=w309:refnum<k20>, "error out"=w308:errorcluster, "Detector de presencia"=w302:bool, "RuedaDetectada1?"=→"RuedaDetectada1?":bool, "RuedaDetectada2?"=→"RuedaDetectada2?":bool)
              n135 = Get Date/Time In Seconds() -> (seconds since 1Jan1904=w304:timestamp)
              n136 = Format Date/Time String(seconds (now)=w304, UTC format=TRUE) -> (date/time string=→"date/time string":string)  [unwired: 1 in]
              n137 = Compound Arithmetic op=OR(w315, w281, w311) -> (w312:bool)
              n138 = case shown="\"STOP_WHD\"" "Developer commad" {
                tunnel: [w329 w330 FALSE ("Adquirir") FALSE ("Adquirir")] -> w288
                tunnel: [FALSE ("Adquirir") w330 w331 w333] -> w287
                frame "Adquirir" {
                  w329 = TRUE ("Adquirir")
                  "Adquirir" <- w329
                }
                frame Default {
                  w330 = FALSE ("Adquirir")
                }
                frame "STOP_WHD" {
                  w331 = TRUE ("Adquirir")
                  "Parar la aplicación" <- w331
                }
                frame "Reset_Controlador" {
                  w333 = TRUE ("Adquirir")
                  "Reset del controlador" <- w333
                }
              }
              "Boton Adquirir?" <- w288
              n139 = xnode "Read/Write Control"("FPGA VI Reference In"=w309, "error in"=w308, "Fotocélula"=w288) -> ("FPGA VI Reference Out"=w299:refnum<k20>, "error out"=w298:errorcluster)
              n140 = Select(t="TEST", s=w312, f="Adquisición") -> (s? t:f=w324:string)
              n141 = Select(t="Configuración", s=w287, f=w324) -> (s? t:f=w292:string)
              n142 = Compound Arithmetic op=OR(w288, w312, w287, w302, "Calibration") -> (w289:bool)
              n143 = Select(t="Calibracion", s="Calibration", f=w292) -> (s? t:f=w285:string)
              n144 = Select(t="UPS", s=w281, f=w285) -> (s? t:f=w282:string)
            }
            n145 = call <vilib>:"Watchdog Clear.vi"("error in (no error)"=w257, "watchdogID in"=w258) -> ("error out"=w256:errorcluster)  [unwired: 5 in]
            n146 = xnode "Read/Write Control"("FPGA VI Reference In"=w251, "error in"=w252) -> ("FPGA VI Reference Out"=w250:refnum<k20>, "error out"=w249:errorcluster, "Direccion 0?"=→"Direccion 0?":bool)
            n147 = Unbundle By Name(w249) -> ("status"=w267:bool)
            n148 = Select(t="TEST", s=w267, f=w268) -> (s? t:f=w263:string)
            n149 = flat-sequence {
              tunnel: [w279] -> w262
              tunnel: w263 -> [w279]
              frame #0 {
                n150 = Get Date/Time In Seconds() -> (seconds since 1Jan1904=w280:timestamp)
                n151 = To Double Precision Float(number=w280) -> (double precision float=→"Tiempo":dbl)
                n152 = local write "Developer commad"("" ("Developer commad")) -> ()
                n153 = local write "Adquirir"(FALSE ("Adquirir")) -> ()
              }
            }
          }
          frame "Adquisición" {
            n154 = flat-sequence {
              tunnel: w340 -> [w380]
              tunnel: w339 -> [w379]
              tunnel: [w380] -> w338
              tunnel: [w379] -> w337
              frame #0 {
                n155 = local read "Report"() -> (w376:string)
                n156 = call "Reporting_datetime.vi"() -> ("String"=w375:string)  [unwired: 11 in]
                n157 = Concatenate Strings(w375, "\nSTATUS: ACQUISITION\nTrain is passing\n\n", w376) -> (w378:string)
                n158 = local write "Report"(w378) -> ()
              }
            }
            n159 = local read "Watchdog config"() -> (w351:T1)
            n160 = call <vilib>:"Watchdog Configure.vi"("error in (no error)"=w350, "expiration actions"=w351, "timeout (1 sec)"=200.0) -> ("error out"=w348:errorcluster, "watchdogID"=w349:u64)  [unwired: 1 in, 2 out]
            n161 = flat-sequence {
              tunnel: w337 -> [w414]
              tunnel: w338 -> [w415]
              tunnel: [w413] -> w365
              tunnel: [w412] -> w364
              tunnel: [w411] -> w363
              tunnel: [w410] -> w362
              tunnel: [w409] -> w361
              tunnel: [w408] -> w360
              tunnel: [w398] -> w353
              tunnel: w349 -> [w397]
              tunnel: w348 -> [w396]
              tunnel: [w397] -> w347
              tunnel: [w396] -> w346
              tunnel: [w430] -> w374
              tunnel: [w447] -> w373
              tunnel: [w446] -> w372
              tunnel: [w445] -> w371
              tunnel: [w438] -> w370
              tunnel: w365 -> [w444]
              tunnel: w364 -> [w443]
              tunnel: w363 -> [w442]
              tunnel: w362 -> [w441]
              tunnel: w361 -> [w440]
              tunnel: w360 -> [w439]
              tunnel: w353 -> [w436]
              tunnel: [w435] -> w352
              tunnel: w347 -> [w434]
              tunnel: w346 -> [w433]
              tunnel: [w431] -> w345
              tunnel: w374 -> [w611]
              tunnel: w373 -> [w606]
              tunnel: w372 -> [w605]
              tunnel: w371 -> [w625]
              tunnel: [w652] -> w357
              tunnel: w370 -> [w654]
              tunnel: [w641] -> w367
              tunnel: [w642] -> w369
              tunnel: [w643] -> w368
              tunnel: w352 -> [w620]
              tunnel: w345 -> [w612]
              tunnel: [w612] -> w343
              tunnel: [w611] -> w342
              frame #0 {
                n162 = local read "Offset_rueda WS 1"() -> (w391:fxp<+/-,24,-4>)
                n163 = local read "Offset_rueda WS 2"() -> (w392:fxp<+/-,24,-4>)
                n164 = local read "Frecuencia de muestreo (Hz)"() -> (w406:dbl)
                n165 = local read "Escaneos de la FIFO por canal"() -> (w395:u32)
                n166 = local read "Canal cero WS1?"() -> (w400:bool)
                n167 = local read "Count(mSec)"() -> (w399:u32)
                n168 = local read "Frecuencia de muestreo y módulo CRIO"() -> (w402:T2)
                n169 = local read "Canal cero WS2"() -> (w390:bool)
                n170 = local read "Digital?"() -> (w401:bool)
                n171 = Get Date/Time In Seconds() -> (seconds since 1Jan1904=→"Inicio pasada":timestamp)
                n172 = local read "Nº de acelerómetros"() -> (w388:i32)
                n173 = local read "Nº inductivos"() -> (w389:i32)
                n174 = xnode "Read/Write Control"("FPGA VI Reference In"=w415, "error in"=w414, "Data Rate"=w402, "Digital?"=w401, "Canal cero WS1?"=w400, "Count(mSec)"=w399, "Offset_WS1"=w391, "Offset_WS2"=w392, "Canal cero WS2?"=w390) -> ("FPGA VI Reference Out"=w405:refnum<k20>, "error out"=w404:errorcluster)
                n175 = local read "RFID LR6 on?"() -> (w393:bool)
                n176 = Add(x=w389, y=w388) -> (x+y=w394:i32)
                n177 = case shown="True" w393 {
                  tunnel: [errorcluster {"status"=FALSE, "code"=0, "source"=""} ("error out") w420] -> w398
                  frame False {
                  }
                  frame True {
                    n178 = local read "RFID_LR6_Error"() -> (w421:errorcluster)
                    n179 = call "LH6HD.vi"("error in (no error)"=w421, "Action"=enum16{"Init", "Start", "Read", "Stop", "Exit"}."Start") -> ("error out"=w420:errorcluster)  [unwired: 8 in, 1 out]
                  }
                }
                n180 = call "DMACalc.vi"("Number of Channels"=w394, "Number of Samples"=w395, "Rate (Hz)"=w406) -> ("Block Size"=w410:u32, "Time to Acquire Block (ms)"=w411:i32, "Host Buffer Size"=w416:u32)  [unwired: 6 in]
                n181 = call "Pathhorafech(SubVI)_varios.vi"("Folder path"=path "c:/Trenes", "Nº de acelerómetros"=w388, "Nº inductivos"=w389) -> ("Acel_Paths"=w384:path[])  [unwired: 1 in, 1 out]
                "Nombre de archivo" <- w384
                n182 = Index Array(array=w384) -> (element=w383:path)  [unwired: 1 in]
                n183 = for {
                  tunnel: w384 -> [w425] mode=indexing
                  tunnel: [w424] -> w409 mode=indexing
                  tunnel: [w423] -> w408
                  n184 = Open/Create/Replace File(file path (use dialog)=w425, operation (0:open)=T5."replace or create", access (0:read/write)=enum16{"read/write", "read-only", "write-only"}."read/write", disable buffering (F)=TRUE) -> (refnum out=w424:refnum<file>, error out=w423:errorcluster)  [unwired: 1 in, 2 out]
                }
                n185 = xnode "Invoke Method"("FPGA VI Reference In"=w405, "error in"=w404, "Requested Depth"=w416) -> ("FPGA VI Reference Out"=w418:refnum<k20>, "error out"=w417:errorcluster)  [unwired: 1 out]
                n186 = local read "Report"() -> (w387:string)
                n187 = Path To String(path=w383) -> (string=w381:string)
                n188 = Concatenate Strings("\nFile created: ", w381, "\n", w387) -> (w386:string)
                n189 = xnode "Invoke Method"("FPGA VI Reference In"=w418, "error in"=w417) -> ("FPGA VI Reference Out"=w413:refnum<k20>, "error out"=w412:errorcluster)
                n190 = local write "Report"(w386) -> ()
              }
              frame #1 {
                n191 = while "Data Acquisition" {
                  tunnel: w444 -> [w498]
                  shift-right: [w522] -> _
                  shift-left: u32 0 ("t") -> [w518]
                  tunnel: w442 -> [w523]
                  tunnel: w441 -> [w521]
                  shift-right: [w524] -> w446
                  shift-left: w443 -> [w515]
                  tunnel: [w519] -> w447
                  tunnel: w440 -> [w502]
                  tunnel: [w503] -> w445
                  shift-right: [w501] -> w438
                  shift-left: w439 -> [w511]
                  stop <- w520 stop-if-true
                  # "Detector de presencia"
                  # "Mide el tiempo de paso del tren y con ello se puede calcular\nla velocidad la unidad"
                  n192 = xnode "Invoke Method"("FPGA VI Reference In"=w498, "error in"=w515, "Number of Elements"=w518, "Timeout (ms)"=0) -> ("FPGA VI Reference Out"=w495:refnum<k20>, "error out"=w500:errorcluster, "Data"=w514:fxp<+/-,24,4>[], "Elements Remaining"=w516:u32)
                  n193 = case "Data Ready" shown="Default" w518 {
                    tunnel: w523 -> [w546 _]
                    tunnel: [w545 u32 0 ("t")] -> w522
                    tunnel: w521 -> [w547 _]
                    tunnel: w516 -> [w544 _]
                    tunnel: w514 -> [_ w569]
                    tunnel: w511 -> [w543 w568]
                    tunnel: [w543 w570] -> w501
                    tunnel: w502 -> [w542 w567]
                    tunnel: [w542 w566] -> w503
                    frame 0 {
                      # "En este caso se compara los elementos que quedan\nen la FIFO del controlador con el tamaño dell bloque\nque aparece en el panel frontal. Si el número de \nelementos en la FIFO es mayor o igual que el tamaño\n del bloque se pasa al siguiente caso y se guardan \nlos datos en un archivo. El reloj que aparece es una\nespera para no consumir recursos."
                      n194 = Greater Or Equal?(x=w544, y=w547) -> (x >= y?=w548:bool)
                      n195 = case shown="False" w548 {
                        tunnel: [u32 0 ("Block Size") w552] -> w545
                        tunnel: [w551 0 ("t")] -> w549
                        tunnel: w546 -> [w551 _]
                        tunnel: w547 -> [_ w552]
                        frame False {
                        }
                        frame True {
                        }
                      }
                      n196 = call "WaitMinTimeBetweenCall.vi"("Minimum ms between calls"=w549) -> ()  [unwired: 2 in]
                    }
                    frame Default {
                      n197 = To Single Precision Float(number=w569) -> (single precision float=w556:sgl[])
                      n198 = Decimate 1D Array(w556) -> (w562:sgl[], w565:sgl[], w564:sgl[], w563:sgl[], w561:sgl[], w560:sgl[], w559:sgl[], w558:sgl[], w557:sgl[], w554:sgl[])
                      n199 = Build Array(w562, w565, w564, w563, w561, w560, w559, w558, w557, w554) -> (w555:sgl[][])
                      n200 = for {
                        tunnel: T6."little-endian" ("byte order (0:big-endian, network order)") -> [w579]
                        shift-right: [w573] -> w570
                        shift-left: w568 -> [w574]
                        tunnel: w555 -> [w577] mode=indexing
                        tunnel: w567 -> [w576] mode=indexing
                        tunnel: [w575] -> w566 mode=indexing
                        n201 = Write to Binary File(file (use dialog)=w576, data=w577, error in=w574, 5:FALSE ("prepend array or string size? (T)"), 9:w579) -> (refnum out=w575:refnum<file>, error out=w573:errorcluster)  [unwired: 2 out]
                      }
                    }
                  }
                  n202 = xnode "Read/Write Control"("FPGA VI Reference In"=w495, "error in"=w500) -> ("FPGA VI Reference Out"=w513:refnum<k20>, "error out"=w512:errorcluster, "Parar"=w491:bool, "Nº Ruedas 1"=→"Nº Ruedas 1":i32, "NºRuedas 2"=→"NºRuedas 2":i32)
                  "Parar" <- w491
                  n203 = case shown="False" w491 {
                    tunnel: [w529 w537] -> w492
                    tunnel: [w530 0.0] -> w506
                    frame False {
                      n204 = local read "Inicio pasada"() -> (w533:timestamp)
                      n205 = Get Date/Time In Seconds() -> (seconds since 1Jan1904=w532:timestamp)
                      n206 = local read "Tiempo de adquisicion"() -> (w525:dbl)
                      n207 = To Double Precision Float(number=w532) -> (double precision float=w531:dbl)
                      n208 = To Double Precision Float(number=w533) -> (double precision float=w534:dbl)
                      n209 = Subtract(x=w531, y=w534) -> (x-y=w530:dbl)
                      "Tiempo de paso (s)" <- w530
                      n210 = local write "Tiempo"(w531) -> ()
                      n211 = local read "Boton Adquirir?"() -> (w526:bool)
                      n212 = Greater?(x=w530, y=w525) -> (0:w528:bool)
                      n213 = Select(t=w528, s=w526, f=FALSE) -> (s? t:f=w529:bool)
                    }
                    frame True {
                      n214 = local read "Tiempo"() -> (w541:dbl)
                      n215 = local read "Tiempo extra al detector de paso (s)"() -> (w536:dbl)
                      n216 = Get Date/Time In Seconds() -> (seconds since 1Jan1904=w538:timestamp)
                      n217 = To Double Precision Float(number=w538) -> (double precision float=w539:dbl)
                      n218 = Subtract(x=w539, y=w541) -> (x-y=w540:dbl)
                      n219 = Greater?(x=w540, y=w536) -> (0:w537:bool)
                    }
                  }
                  "Fin" <- w492
                  n220 = local read "Timeout ruedas"() -> (w490:dbl)
                  n221 = xnode ("CheckLate")("FPGA VI Reference In"=w513, "error in"=w512) -> ("FPGA VI Reference Out"=w497:refnum<k20>, "error out"=w508:errorcluster, "Buffer Underflow"=→"Buffer Underflow":bool, "Buffer Overflow"=w499:bool)
                  "Buffer Overflow" <- w499
                  n222 = Greater?(x=w506, y=w490) -> (0:w504:bool)
                  "Timeout ruedas" <- w504
                  n223 = call "ErrorOverFlow.vi"("Buffer Overflow"=w499) -> ("error out"=w507:errorcluster)
                  n224 = Merge Errors(w508, w507) -> (w496:errorcluster)
                  n225 = Unbundle By Name(w501) -> ("status"=w505:bool)
                  n226 = Unbundle By Name(w496) -> ("status"=w510:bool)
                  n227 = Compound Arithmetic op=OR(w510, w492, w504, w505) -> (w520:bool)
                  "result" <- w520
                  n228 = case "Flush" shown="True" w520 {
                    tunnel: [w580 w585] -> w524
                    tunnel: [w581 w584] -> w519
                    tunnel: w497 -> [w581 w583]
                    tunnel: w496 -> [w580 w582]
                    frame False {
                    }
                    frame True {
                      n229 = xnode "Invoke Method"("FPGA VI Reference In"=w583, "error in"=w582) -> ("FPGA VI Reference Out"=w584:refnum<k20>, "error out"=w585:errorcluster)
                    }
                  }
                  "Block Size" <- w521
                  "Time to Acquire Block (ms)" <- w523
                }
                n230 = call <vilib>:"Watchdog Whack.vi"("error in (no error)"=w433, "reset watchdog after expire? (F)"=TRUE, "watchdogID in"=w434) -> ("error out"=w430:errorcluster, "watchdogID out"=w431:u64)  [unwired: 2 in, 1 out]
                n231 = local read "RFID LR6 on?"() -> (w429:bool)
                n232 = case shown="True" w429 {
                  tunnel: w436 -> [w448 w454]
                  tunnel: [w448 w453] -> w435
                  frame False {
                  }
                  frame True {
                    n233 = while {
                      shift-right: [w461] -> w453
                      shift-left: w454 -> [w462]
                      shift-right: [w460] -> w451
                      shift-left: string[] [] -> [w459]
                      shift-right: [w455] -> w449
                      shift-left: i32[] [] -> [w456]
                      i -> [w457]
                      stop <- w458 stop-if-true
                      n234 = case shown="No Error" w462 {
                        selector: w462 -> [w473 _]
                        tunnel: [w472 w488] -> w461
                        tunnel: [w468 string[] []] -> w460
                        tunnel: w459 -> [w467 _]
                        tunnel: w457 -> [w466 _]
                        tunnel: w456 -> [w465 _]
                        tunnel: [w464 i32[] []] -> w455
                        frame No Error {
                          n235 = call "LH6HD.vi"("error in (no error)"=w473, "Action"=enum16{"Init", "Start", "Read", "Stop", "Exit"}."Read") -> ("error out"=w472:errorcluster, "Tag"=w469:string)  [unwired: 8 in]
                          n236 = Not Equal?(x="", y=w469) -> (x != y?=w470:bool)
                          n237 = case shown="False" w470 {
                            tunnel: w469 -> [_ w482]
                            tunnel: [w476 w481] -> w468
                            tunnel: w467 -> [w476 w480]
                            tunnel: w466 -> [_ w477]
                            tunnel: w465 -> [w475 w479]
                            tunnel: [w475 w478] -> w464
                            frame False {
                            }
                            frame True {
                              n238 = Build Array (concatenate)(w480, w482) -> (w481:string[])
                              n239 = Build Array (concatenate)(w479, w477) -> (w478:i32[])
                            }
                          }
                        }
                        frame Error {
                          n240 = local read "LR6 IP address"() -> (w485:string)
                          n241 = local read "DeviceAddress"() -> (w483:u8)
                          n242 = local read "Port LR6"() -> (w486:u16)
                          n243 = call "LH6HD.vi"("DeviceAddress"=w483, "Reader Port"=w486, "IP Address"=w485, "Action"=enum16{"Init", "Start", "Read", "Stop", "Exit"}."Init") -> ("error out"=w488:errorcluster)  [unwired: 6 in, 1 out]
                        }
                      }
                      n244 = Wait Until Next ms Multiple(millisecond multiple=u32 500) -> ()  [unwired: 1 out]
                      n245 = local read "result"() -> (w458:bool)
                      "it-LR6" <- w457
                    }
                    "TAGs LR6" <- w451
                    "it-read-LR6" <- w449
                  }
                }
              }
              frame #2 {
                n246 = local read "RFID LR6 on?"() -> (w607:bool)
                n247 = Array Size(array=w625) -> (size(s)=w623:i32)
                n248 = local read "timeout ms (60000)"() -> (w610:i32)
                n249 = local read "AURA wheel test"() -> (w587:bool)
                n250 = case shown="True" w607 {
                  tunnel: w620 -> [w660 w666]
                  tunnel: [w660 w661] -> w619
                  frame False {
                  }
                  frame True {
                    n251 = call "LH6HD.vi"("error in (no error)"=w666, "Action"=enum16{"Init", "Start", "Read", "Stop", "Exit"}."Stop") -> ("error out"=w661:errorcluster)  [unwired: 8 in, 1 out]
                    n252 = call "Reporting_error.vi"("error out 2"=w661, "Concept"="Active RFID") -> ("Reporting"=w663:string)  [unwired: 1 in]
                    n253 = local read "Report"() -> (w664:string)
                    n254 = Concatenate Strings(w663, w664) -> (w662:string)
                    n255 = local write "Report"(w662) -> ()
                  }
                }
                n256 = local read "bytes to read"() -> (w609:i32)
                n257 = local read "RFID NEM on?"() -> (w608:bool)
                n258 = Decrement(x=w623) -> (x-1=w624:i32)
                n259 = local read "Puerto RFID"() -> (w640:u16)
                n260 = local read "RFID_Error"() -> (w650:errorcluster)
                n261 = local read "IP RFID"() -> (w622:string)
                n262 = local read "RFID_ID"() -> (w649:refnum<k5>)
                n263 = Index Array(array=w625, index=w624) -> (element=w633:refnum<file>)
                n264 = local write "result"(FALSE ("result")) -> ()
                n265 = xnode "Read/Write Control"("FPGA VI Reference In"=w606, "error in"=w605) -> ("FPGA VI Reference Out"=w651:refnum<k20>, "error out"=w602:errorcluster, "Chassis Temperature"=w659:i16)
                n266 = local read "TAGs LR6"() -> (w589:string[])
                n267 = case shown="True" w608 {
                  tunnel: w650 -> [w669 w682]
                  tunnel: w649 -> [w668 w681]
                  tunnel: [w668 w680] -> w648
                  tunnel: [w669 w670] -> w644
                  tunnel: w640 -> [_ w679]
                  tunnel: w622 -> [_ w678]
                  tunnel: [_ w677] -> w604
                  tunnel: w610 -> [_ w676]
                  tunnel: w609 -> [_ w675]
                  frame False {
                  }
                  frame True {
                    n268 = call "RFID_28_03_12.vi"("BYTES TO READ"=w675, "TIMEOUT"=w676, "RFID_Error"=w682, "Puerto RFID"=w679, "IP RFID"=w678, "RFID ID"=w681) -> ("RFID Error"=w670:errorcluster, "connection ID out"=w680:refnum<k5>, "TAGs HEX"=w677:string[])  [unwired: 1 in, 1 out]
                    n269 = call "Reporting_error.vi"("error out 2"=w670, "Concept"="Passive RFID") -> ("Reporting"=w672:string)  [unwired: 1 in]
                    n270 = local read "Report"() -> (w673:string)
                    n271 = Concatenate Strings(w672, w673) -> (w671:string)
                    n272 = local write "Report"(w671) -> ()
                  }
                }
                "TAGs HEX" <- w604
                n273 = Select(t=string[] ["A0000000000000000TESTNEM7", "A0000000000000000TESTNEM8"], s=w587, f=w589) -> (s? t:f=w586:string[])
                n274 = Divide(x=w659, y=4.0) -> (x/y=w598:dbl)
                "Temperatura (ºC)" <- w598
                n275 = local read "Tiempo de paso (s)"() -> (w646:dbl)
                n276 = for {
                  tunnel: w586 -> [w685] mode=indexing
                  tunnel: [w683] -> w613 mode=indexing
                  n277 = Search and Replace String(input string=w685, search string="00") -> (result string=w683:string)  [unwired: 6 in, 3 out]
                }
                n278 = local write "RFID_LR6_Error"(w619) -> ()
                n279 = Index Array(array=w604) -> (element=w618:string)  [unwired: 1 in]
                n280 = local read "Nº Ruedas 1"() -> (w596:i32)
                n281 = local read "NºRuedas 2"() -> (w600:i32)
                n282 = Not Equal?(x=w618, y="" ("delimiter (\\t)")) -> (x != y?=w616:bool)
                "Plataformas?" <- w616
                n283 = Multiply(x=w646, y=1000.0) -> (x*y=w597:dbl)
                n284 = case shown="True" w616 {
                  tunnel: w613 -> [w686 w687]
                  tunnel: [w686 w689] -> w599
                  tunnel: w604 -> [_ w688]
                  frame False {
                  }
                  frame True {
                    n285 = call "Union_TAGs_RFIDs.vi"("TAGs LR6"=w687, "TAGs HEX"=w688) -> ("TAGs"=w689:string[])
                  }
                }
                "TAGs" <- w599
                n286 = local write "RFID_ID"(w648) -> ()
                n287 = local write "RFID_Error"(w644) -> ()
                n288 = Build Array(w598, w597, w596, w600) -> (w601:dbl[])
                n289 = Build Array(w598, w597, w596) -> (w595:dbl[])
                n290 = local read "Direccion 0?"() -> (w594:bool)
                n291 = local read "Nombre de archivo"() -> (w632:path[])
                n292 = for {
                  shift-right: [w695] -> w638
                  shift-left: string[] [] -> [w694]
                  tunnel: w599 -> [w693] mode=indexing
                  n293 = Insert Into Array(array=w694, new element=w693) -> (w695:string[])  [unwired: 1 in]
                }
                n294 = Bundle("error out"=w602, w601, "TAGs"=w599, "Direccion 0?"=w594) -> (w593:T11)  [unwired: 1 in]
                n295 = Delete From Array(array=w632) -> (deleted portion=w631:path)  [unwired: 2 in, 1 out]
                n296 = To Single Precision Float(number=w595) -> (single precision float=w657:sgl[])
                n297 = xnode "Read/Write Control"("FPGA VI Reference In"=w651, "error in"=w602, "Stop"=TRUE ("stop")) -> ("FPGA VI Reference Out"=w635:refnum<k20>, "error out"=w634:errorcluster)
                n298 = call "Reporting_acqu.vi"("output cluster"=w593, "address repoting"=path "C:/Reporting/Reporting_adqu.txt" ("file (use dialog)")) -> ("Reporting"=w590:string)  [unwired: 1 in]
                n299 = Path To String(path=w631) -> (string=w637:string)
                n300 = local read "Report"() -> (w591:string)
                n301 = Write to Binary File(file (use dialog)=w633, data=w657, error in=w654, 5:FALSE ("prepend array or string size? (T)"), 9:T6."little-endian" ("byte order (0:big-endian, network order)")) -> (error out=w630:errorcluster)  [unwired: 3 out]
                n302 = local read "Timeout ruedas"() -> (w647:bool)
                n303 = Build Array (concatenate)(w637, w638) -> (w614:string[])
                n304 = local read "TAGS leidos"() -> (w626:path)
                n305 = Concatenate Strings(w590, w591) -> (w592:string)
                n306 = for {
                  shift-right: [w692] -> w641
                  shift-left: w630 -> [w691]
                  tunnel: w625 -> [w690] mode=indexing
                  n307 = Close File(refnum=w690, error in=w691) -> (error out=w692:errorcluster)  [unwired: 1 out]
                }
                n308 = local write "Report"(w592) -> ()
                n309 = xnode "Invoke Method"("FPGA VI Reference In"=w635, "error in"=w634) -> ("FPGA VI Reference Out"=w643:refnum<k20>, "error out"=w642:errorcluster)
                n310 = call-poly <vilib>:"Write Delimited Spreadsheet.vi"("file path (dialog if empty)"=w626, "1D data"=w614, "append to file? (new file:F)"=TRUE ("transpose? (no:F)"), "transpose? (no:F)"=TRUE ("append to file? (new file:F)"), "delimiter (\\t)"=";" ("delimiter (\\t)")) -> ()  [unwired: 9 in, 2 out]
                n311 = Select(t="TEST", s=w647, f="Procesado") -> (s? t:f=w652:string)
              }
            }
            n312 = call <vilib>:"Watchdog Clear.vi"("error in (no error)"=w342, "watchdogID in"=w343) -> ("error out"=w344:errorcluster)  [unwired: 5 in]
            n313 = Unbundle By Name(w369) -> ("status"=w358:bool)
            n314 = Unbundle By Name(w367) -> ("status"=w359:bool)
            n315 = Merge Errors(w367, w344) -> (w366:errorcluster)
            n316 = Compound Arithmetic op=OR(w358, w359) -> (w356:bool)
            n317 = Select(t="TEST", s=w356, f=w357) -> (s? t:f=w354:string)
          }
          frame "Procesado" {
            n318 = flat-sequence {
              tunnel: w701 -> [w720]
              tunnel: [w720] -> w700
              tunnel: w699 -> [w716]
              tunnel: [w716] -> w698
              frame #0 {
                n319 = local read "Report"() -> (w717:string)
                n320 = call "Reporting_datetime.vi"() -> ("String"=w715:string)  [unwired: 11 in]
                n321 = Concatenate Strings(w715, "\nSTATUS: PROCESSING\nProcessing the measurement\n\n", w717) -> (w719:string)
                n322 = local write "Report"(w719) -> ()
              }
            }
            n323 = local read "Watchdog config"() -> (w707:T1)
            n324 = call <vilib>:"Watchdog Configure.vi"("error in (no error)"=w710, "expiration actions"=w707, "timeout (1 sec)"=300.0) -> ("error out"=w709:errorcluster, "watchdogID"=w706:u64)  [unwired: 1 in, 2 out]
            n325 = flat-sequence {
              tunnel: w709 -> [w727]
              tunnel: w706 -> [w723]
              tunnel: [w722] -> w705
              tunnel: [w721] -> w704
              tunnel: [w938] -> w703
              tunnel: w705 -> [w938]
              tunnel: [w937] -> w702
              tunnel: w704 -> [w937]
              frame #0 {
                n326 = flat-sequence {
                  tunnel: [w799] -> w729
                  tunnel: [w785] -> w728
                  tunnel: w727 -> [w766]
                  tunnel: [w748] -> w724
                  tunnel: [w787] -> w726
                  tunnel: [w739] -> w725
                  tunnel: w723 -> [w767]
                  tunnel: [w764] -> w722
                  tunnel: [w763] -> w721
                  frame #0 {
                    n327 = local read "AURA wheel test"() -> (w737:bool)
                    n328 = case shown="True" w737 {
                      tunnel: [w802 w803] -> w736
                      tunnel: [w801 path[] [path "c:/Trenes_prueba/A_0_TEST.bin", path "c:/Trenes_prueba/A_1_TEST.bin", path "c:/Trenes_prueba/A_2_TEST.bin", path "c:/Trenes_prueba/A_3_TEST.bin", path "c:/Trenes_prueba/A_4_TEST.bin", path "c:/Trenes_prueba/A_5_TEST.bin", path "c:/Trenes_prueba/A_6_TEST.bin", path "c:/Trenes_prueba/A_7_TEST.bin", path "c:/Trenes_prueba/I_0_TEST.bin", path "c:/Trenes_prueba/I_1_TEST.bin"]] -> w735
                      frame False {
                        n329 = local read "Nombre de archivo"() -> (w801:path[])
                        n330 = local read "TAGs"() -> (w802:string[])
                      }
                      frame True {
                        w803 = string[] ["A0000000000000000TESTNEM7", "A0000000000000000TESTNEM8"]
                        n331 = local write "TAGs LR6"(w803) -> ()
                      }
                    }
                    n332 = local read "Tabla_flota"() -> (w784:string[][])
                    n333 = call <vilib>:"Watchdog Whack.vi"("error in (no error)"=w766, "reset watchdog after expire? (F)"=TRUE, "watchdogID in"=w767) -> ("error out"=w763:errorcluster, "watchdogID out"=w764:u64)  [unwired: 2 in, 1 out]
                    n334 = local read "Puntos medios de las ventanas"() -> (w786:dbl[][])
                    n335 = call "Series_ejes_flota.vi"("Tabla_flota"=w784, "Tags"=w736) -> ("Nº Ejes"=w761:i32[], "Series del convoy"=w778:string[])  [unwired: 2 in, 1 out]
                    "Nº Ejes" <- w761
                    n336 = Array Size(array=w735) -> (size(s)=w793:i32)
                    n337 = Add Array Elements(numeric array=w761) -> (sum=w747:i32)
                    "Ejes_convoy" <- w747
                    n338 = Subtract(x=w793, y=2 ("length")) -> (x-y=w795:i32)
                    n339 = Array Size(array=w778) -> (size(s)=→"Nº UTs":i32)
                    n340 = local read "Series_flota"() -> (w783:string[])
                    n341 = Delete From Array(array=w735, length=2, index=w795) -> (deleted portion=w768:path[], array with subset deleted=w787:path[])
                    n342 = Index Array(array=w768) -> (element #2=w762:path)  [unwired: 2 in, 1 out]
                    n343 = call "Distancias_ejes_convoy.vi"("Series_flota1"=w778, "Ejes_UT"=w761, "Puntos medios de las ventanas"=w786, "Series_flota"=w783) -> ("Distancias_entre_ejes_convoy"=w785:dbl[])  [unwired: 1 in]
                    n344 = Read from Binary File(5:sgl 0.0, 9:T6."little-endian" ("byte order (0:big-endian, network order)"), 10:-1 ("count (1)"), 11:w762) -> (0:w791:errorcluster, 2:w770:sgl[], 3:w792:refnum<file>)  [unwired: 1 in, 2 out]
                    n345 = local read "Frecuencia de muestreo (Hz)"() -> (w752:dbl)
                    n346 = local read "Offset_rueda WS 2"() -> (w753:fxp<+/-,24,-4>)
                    n347 = local read "it-LR6"() -> (w773:i32)
                    n348 = local read "it-read-LR6"() -> (w774:i32[])
                    n349 = local read "Plataformas?"() -> (w772:bool)
                    n350 = local read "TAGs"() -> (w776:string[])
                    n351 = local read "TAGs LR6"() -> (w775:string[])
                    n352 = Close File(refnum=w792, error in=w791) -> (error out=w731:errorcluster)  [unwired: 1 out]
                    n353 = Array Size(array=w770) -> (size(s)=w782:i32)
                    n354 = Subtract(x=w782, y=3 ("length")) -> (x-y=w780:i32)
                    n355 = Delete From Array(array=w770, length=3, index=w780) -> (array with subset deleted=w759:sgl[])  [unwired: 1 out]
                    n356 = call "TAGs_AURAwheel.vi"("Nº Ejes"=w761, "TAGs"=w776, "Ejes_convoy"=w747, "it-LR6"=w773, "TAGs LR6"=w775, "it-read-LR6"=w774, "Plataformas?"=w772) -> ("TAGS_AURA"=→"TAGs_AURAwheel":string[][])  [unwired: 1 in]
                    n357 = call "Analogico_digital.vi"("Array"=w759, "Offset WS"=w753, "Frecuencia muestreo"=w752) -> ("array w/ subset deleted"=w754:sgl[], "Tiempo\npaso"=w751:dbl)  [unwired: 6 in]
                    n358 = call "Puntos medio de pulso.vi"("DI Inductivo"=w754) -> ("Puntos"=w799:sgl[], "Número de ejes"=w741:i32)  [unwired: 1 in]
                    "Número de ejes detectados" <- w741
                    n359 = disable-structure shown="Disabled" {
                      disable-tunnel: w759 -> [w811 w814]
                      disable-tunnel: [FALSE ("element") TRUE ("element")] -> w756
                      disable-tunnel: [w805 w813] -> w755
                      frame Disabled {
                        n360 = Equal?(x=w811, y=0.0) -> (x = y?=w808:bool[])
                        n361 = Equal?(x=w811, y=1.0) -> (x = y?=w809:bool[])
                        n362 = Or(x=w808, y=w809) -> (x .or. y?=w805:bool[])
                      }
                      frame Enabled {
                        n363 = Greater?(x=w814, y=0.1) -> (0:w813:bool[])
                      }
                    }
                    n364 = Decrement(x=w741) -> (x-1=w798:i32)
                    n365 = call "Reporting_error.vi"("error out 2"=w731, "Concept"="Measurement reading") -> ("Reporting"=w733:string)  [unwired: 1 in]
                    n366 = Get Volume Info(11:path "c:/" ("path")) -> (1:w742:i64)  [unwired: 1 in, 5 out]
                    "Disco Duro Disponible (bytes)" <- w742
                    n367 = local read "Report"() -> (w734:string)
                    n368 = call "Calculo_Velocidad.vi"("Tiempo de paso (s)"=w751, "Ejes"=w798, "Puntos iniciales de las ventanas"=w785) -> ("V (m/s)"=→"V (m/s)":dbl, "Longitud de la unidad"=→"Longitud de la unidad":dbl)
                    n369 = Concatenate Strings(w733, w734) -> (w732:string)
                    n370 = Equal?(x=w747, y=w741) -> (x = y?=w739:bool)
                    n371 = Not Equal?(x=w741, y=0) -> (x != y?=w738:bool)
                    n372 = Search 1D Array(1D array=w755, element=w756) -> (index of element=w757:i32)  [unwired: 1 in]
                    n373 = local write "Report"(w732) -> ()
                    n374 = Build Array(w747, w741, w742) -> (w746:i64[])
                    n375 = Equal?(x=w757, y=-1) -> (x = y?=w760:bool)
                    n376 = Compound Arithmetic op=AND(w739, w738, w760) -> (w748:bool)
                    "Archivo\nvalido?" <- w748
                    n377 = Bundle(w746, w748) -> (w744:cluster{i64[], bool})  [unwired: 1 in]
                    n378 = call "Reporting_proc.vi"("output cluster 2"=w744, "address repoting"=path "C:/Reporting/Reporting_proc.txt" ("file (use dialog)")) -> ("Reporting"=w743:string)  [unwired: 1 in]
                    n379 = local read "Report"() -> (w749:string)
                    n380 = Concatenate Strings(w743, w749) -> (w750:string)
                    n381 = local write "Report"(w750) -> ()
                  }
                }
                n382 = case shown="False" w724 {
                  tunnel: w729 -> [_ w849]
                  tunnel: w728 -> [_ w847]
                  tunnel: w726 -> [_ w848]
                  tunnel: w725 -> [w816 _]
                  frame False {
                    n383 = local read "Nombre de archivo"() -> (w817:path[])
                    n384 = for {
                      tunnel: w817 -> [w819] mode=indexing
                      tunnel: w816 -> [w818]
                      n385 = flat-sequence {
                        tunnel: w819 -> [w829]
                        tunnel: [w829] -> w822
                        tunnel: [w828] -> w821
                        tunnel: w818 -> [w827]
                        tunnel: w822 -> [w836]
                        tunnel: [w835] -> w820
                        tunnel: w821 -> [w835]
                        tunnel: w820 -> [w838]
                        frame #0 {
                          w828 = path "c:/Est_Adq.csv" ("file path (use dialog)")
                          n386 = Path To String(path=w829) -> (string=w830:string)
                          n387 = Select(t="Nº Ejes detectados WS diferente a Nº Ejes TAGs" ("delimiter (\\t)"), s=w827, f="La señal del inductivo no es digital" ("delimiter (\\t)")) -> (s? t:f=w824:string)
                          n388 = Build Array(w830, w824) -> (w823:string[])
                          n389 = call-poly <vilib>:"Write Delimited Spreadsheet.vi"("file path (dialog if empty)"=w828, "1D data"=w823, "append to file? (new file:F)"=FALSE ("transpose? (no:F)"), "transpose? (no:F)"=TRUE ("append to file? (new file:F)"), "delimiter (\\t)"=";" ("delimiter (\\t)")) -> ()  [unwired: 9 in, 2 out]
                        }
                        frame #1 {
                          n390 = local read "Borrar archivos\nadquisicion con error"() -> (w834:bool)
                          n391 = case shown="True" w834 {
                            tunnel: w836 -> [_ w837]
                            frame False {
                            }
                            frame True {
                              n392 = Delete(path (use dialog)=w837) -> ()  [unwired: 1 in, 6 out]
                            }
                          }
                        }
                        frame #2 {
                          n393 = File/Directory Info(path=w838) -> (size=w841:i64)  [unwired: 1 in, 6 out]
                          n394 = Greater?(x=w841, y=i64 1000000) -> (0:w839:bool)
                          n395 = case shown="True" w839 {
                            tunnel: w838 -> [_ w842]
                            frame False {
                            }
                            frame True {
                              n396 = Delete(path (use dialog)=w842) -> ()  [unwired: 4 in, 3 out]
                            }
                          }
                        }
                      }
                    }
                  }
                  frame True {
                    n397 = flat-sequence {
                      tunnel: w849 -> [w926]
                      tunnel: w848 -> [w923]
                      tunnel: w847 -> [w927]
                      tunnel: [w910] -> w846
                      frame #0 {
                        # "SALIDA \n\nMáximos por rueda inductivo"
                        # "8 acelerómetros"
                        # "Velocidad"
                        n398 = local read "Frecuencia de muestreo (Hz)"() -> (w925:dbl)
                        n399 = local read "Distancia de acelerómetros"() -> (w915:dbl[])
                        n400 = local read "Parámetros acelerómetros"() -> (w922:dbl[])
                        n401 = local read "Número de ejes detectados"() -> (w921:i32)
                        n402 = local read "Distancias generales"() -> (w920:dbl[])
                        n403 = local read "dt RMS"() -> (w924:dbl)
                        n404 = local read "Direccion 0?"() -> (w912:bool)
                        n405 = Index Array(array=w920, index=1) -> (element=w918:dbl)
                        n406 = Select(t=0.0, s=w912, f=w918) -> (s? t:f=w916:dbl)
                        n407 = Subtract(x=w916, y=w915) -> (x-y=w914:dbl[])
                        n408 = Absolute Value(x=w914) -> (abs(x)=w913:dbl[])
                        n409 = call "Procesado_aRMS_BIdirecc.vi"("Paths_canales_aRMS"=w923, "Ejes Procesados"=w921, "Distancias\nacelerometros"=w913, "Distancias generales (m)"=w920, "Distancias centrales de las ruedas\n               configuración (m)"=w927, "Frecuencia de muestreo"=w925, "Parámetros acelerómetros"=w922, "dt RMS 2"=w924, "Puntos"=w926) -> ("Max RMS Ruedas"=w911:dbl[][])  [unwired: 2 in]
                        n410 = Transpose 2D Array(2D array=w911) -> (transposed array=w910:dbl[][])
                        "Max RMS Ruedas" <- w910
                        n411 = call "Reporting_proc_RMS.vi"("Max RMS Ruedas"=w910) -> ("String"=w908:string)
                        n412 = local read "Report"() -> (w909:string)
                        n413 = Concatenate Strings(w908, w909) -> (w907:string)
                        n414 = local write "Report"(w907) -> ()
                      }
                    }
                    n415 = local read "Use Aura?"() -> (w845:bool)
                    n416 = local read "TAGs_AURAwheel"() -> (w844:string[][])
                    n417 = local read "Nº Ejes"() -> (w843:i32[])
                    n418 = for {
                      tunnel: w845 -> [w853]
                      tunnel: w844 -> [w852] mode=indexing
                      shift-right: [w851] -> _
                      shift-left: w846 -> [w854]
                      tunnel: w843 -> [w850] mode=indexing
                      # "dev.api.aurawheel.com"
                      n419 = case shown="True" w853 {
                        tunnel: w854 -> [w855 w874]
                        tunnel: w852 -> [_ w875]
                        tunnel: [w855 w873] -> w851
                        tunnel: w850 -> [_ w871]
                        frame False {
                        }
                        frame True {
                          w859 = "\n"
                          w882 = cluster{"status":string} {"status"=""}
                          n420 = local read "Parametros AuraWheel"() -> (w906:string[])
                          n421 = Delete From Array(array=w874, length=w871, index (row)=0) -> (deleted portion=w870:dbl[][], array with subset deleted=w873:dbl[][])  [unwired: 1 in]
                          n422 = Get Date/Time In Seconds() -> (seconds since 1Jan1904=w903:timestamp)
                          n423 = Format Date/Time String(time format string (%c)="%H:%M:%S%3u", seconds (now)=w903) -> (date/time string=w901:string)  [unwired: 1 in]
                          n424 = Get Date/Time In Seconds() -> (seconds since 1Jan1904=w878:timestamp)
                          n425 = Scan From String(format string="%d:%d:%f", input string=w901) -> (output 1=w898:i32, output 2=w897:i32, output 3=w895:dbl)  [unwired: 5 in, 3 out]
                          n426 = local read "V (m/s)"() -> (w866:dbl)
                          n427 = local read "Temperatura (ºC)"() -> (w876:dbl)
                          n428 = Multiply(x=w866, y=3.6) -> (x*y=w864:dbl)
                          n429 = Multiply(x=w895, y=1000.0) -> (x*y=w891:dbl)
                          n430 = call "Time_to_ms.vi"("seconds since 1Jan1904"=w878) -> ("Numeric"=w877:dbl)  [unwired: 1 in]
                          n431 = Multiply(x=w897, y=60000) -> (x*y=w892:i32)
                          n432 = Multiply(x=3600000, y=w898) -> (x*y=w893:i32)
                          n433 = Index Array(array=w906) -> (element #1=w869:string, element #2=w868:string, element #3=w867:string)  [unwired: 3 in]
                          n434 = call "aw_WRDCluster_8acel.vi"("Array TAGs"=w875, "Max RMS Ruedas"=w870, "TimeStamp"=w877, "p_sp"=w864, "p_tp"=w876) -> ("JSON cluster"=w904:T12)  [unwired: 1 in]
                          n435 = Compound Arithmetic op=ADD(w893, w892, w891) -> (w890:dbl)
                          n436 = To Variant(anything=w904) -> (Variant=w887:variant)
                          n437 = To Unsigned Long Integer(number=w890) -> (unsigned 32bit integer=w889:u32)
                          n438 = call "gjson_Create.vi"("JSON Object in"=w887) -> ("error out"=w885:errorcluster, "JSON String Out"=w886:string)  [unwired: 9 in]
                          n439 = Number To Decimal String(number=w889) -> (decimal integer string=w888:string)  [unwired: 1 in]
                          n440 = To Variant(anything=w882) -> (Variant=w881:variant)
                          n441 = call "aw_SendData.vi"("pwd"=w869, "x-nem-datetime"=w888, "User"=w868, "error in"=w885, "JSON Object"=w886, "URL"=w867) -> ("error out"=w883:errorcluster, "Response JSON"=w884:string, "Response headers"=w860:string)  [unwired: 3 in]
                          "Response headers" <- w860
                          n442 = call "gjson_Parse.vi"("error in"=w883, "JSON String In"=w884, "JSON Cluster"=w881) -> ("error out"=w879:errorcluster, "JSON Cluster Out"=w880:variant)  [unwired: 7 in]
                          n443 = Variant To Data(error in=w879, type=w882, Variant=w880) -> (data=→"data":cluster{"status":string}, error out=w861:errorcluster)
                          "error AURA" <- w861
                          n444 = local read "Report"() -> (w857:string)
                          n445 = call "Reporting_error.vi"("error out 2"=w861, "Concept"="A.U.R.A. Wheel Connection") -> ("Reporting"=w862:string)  [unwired: 1 in]
                          n446 = Concatenate Strings(w862, w859, w859, w860, w859) -> (w858:string)
                          "Report_AURA" <- w858
                          n447 = Concatenate Strings(w858, w857) -> (w856:string)
                          n448 = local write "Report"(w856) -> ()
                        }
                      }
                    }
                  }
                }
              }
              frame #1 {
                n449 = local read "Archivo\nvalido?"() -> (w934:bool)
                n450 = local read "Report_AURA"() -> (w931:string)
                n451 = local read "Bytes libre despues de borrar"() -> (w935:u32)
                n452 = local read "Max archivos"() -> (w932:u32)
                n453 = local read "Path LOG"() -> (w933:path)
                n454 = local read "LOG.txt"() -> (w928:path)
                n455 = local read "Report"() -> (w930:string)
                n456 = local read "Bytes min libre"() -> (w936:u32)
                n457 = local read "TAGS leidos"() -> (w939:path)
                n458 = File/Directory Info(path=w939) -> (size=w942:i64)  [unwired: 1 in, 6 out]
                n459 = case shown="True" w934 {
                  frame False {
                  }
                  frame True {
                    n460 = local read "Nombre de archivo"() -> (w944:path[])
                    n461 = call "Comprimir_a_1_archivo.vi"("Acel_paths"=w944) -> ("path_Pasada"=→"created path":path)
                  }
                }
                n462 = Greater?(x=w942, y=i64 1000000) -> (0:w940:bool)
                n463 = case shown="True" w940 {
                  tunnel: w939 -> [_ w945]
                  frame False {
                  }
                  frame True {
                    n464 = Delete(path (use dialog)=w945) -> ()  [unwired: 4 in, 3 out]
                  }
                }
                n465 = call "BORRADO_MEJORADO_Gonzalo.vi"("Bytes LIBRE OK"=w935, "Bytes Minimo de Memoria libre"=w936) -> ()  [unwired: 10 in]
                n466 = call "Saving_LOG.vi"("Path"=w928, "Report"=w930, "Report AURA"=w931, "Path Carpeta"=w933, "Nº Archivos Max"=w932) -> ("Report"=w929:string)  [unwired: 9 in, 1 out]
                n467 = local write "Report"(w929) -> ()
              }
            }
            n468 = call <vilib>:"Watchdog Clear.vi"("error in (no error)"=w702, "watchdogID in"=w703) -> ("error out"=w696:errorcluster)  [unwired: 5 in]
            n469 = Merge Errors(w698, w696) -> (w714:errorcluster)
            n470 = Unbundle By Name(w714) -> ("status"=w712:bool)
            n471 = Select(t="TEST", s=w712, f="Espera") -> (s? t:f=w711:string)
          }
          frame "TEST" {
            n472 = flat-sequence {
              tunnel: w950 -> [w967]
              tunnel: [w967] -> w948
              frame #0 {
                n473 = local read "Report_AURA"() -> (w963:string)
                n474 = local read "Max archivos"() -> (w964:u32)
                n475 = call "Reporting_datetime.vi"() -> ("String"=w966:string)  [unwired: 11 in]
                n476 = local read "Path LOG"() -> (w965:path)
                n477 = local read "LOG.txt"() -> (w960:path)
                n478 = local read "Report"() -> (w962:string)
                n479 = local read "Report"() -> (w968:string)
                n480 = Concatenate Strings(w966, "\nSTATUS: ERROR TEST\n\n", w968) -> (w970:string)
                n481 = call "Saving_LOG.vi"("Path"=w960, "Report"=w962, "Report AURA"=w963, "Path Carpeta"=w965, "Nº Archivos Max"=w964) -> ("Report"=w961:string)  [unwired: 9 in, 1 out]
                n482 = local write "Report"(w970) -> ()
                n483 = local write "Report"(w961) -> ()
              }
            }
            n484 = local read "Watchdog config"() -> (w955:T1)
            n485 = call <vilib>:"Watchdog Configure.vi"("error in (no error)"=w946, "expiration actions"=w955, "timeout (1 sec)"=200.0) -> ("error out"=w956:errorcluster, "watchdogID"=w953:u64)  [unwired: 1 in, 2 out]
            n486 = Merge Errors(w948, w946) -> (w947:errorcluster)
            n487 = flat-sequence {
              tunnel: [w980] -> w959
              tunnel: w956 -> [w975]
              tunnel: w947 -> [w993]
              tunnel: [w976] -> w957
              tunnel: w953 -> [w974]
              tunnel: [w973] -> w952
              tunnel: [w972] -> w951
              frame #0 {
                n488 = call <vilib>:"Watchdog Whack.vi"("error in (no error)"=w975, "reset watchdog after expire? (F)"=TRUE, "watchdogID in"=w974) -> ("error out"=w972:errorcluster, "watchdogID out"=w973:u64)  [unwired: 2 in, 1 out]
                n489 = Get Date/Time In Seconds() -> (seconds since 1Jan1904=w987:timestamp)
                n490 = local read "Ultimo TEST"() -> (w988:timestamp)
                n491 = To Double Precision Float(number=w987) -> (double precision float=w989:dbl)
                n492 = Subtract(x=w989, y=3600.0) -> (x-y=w991:dbl)
                n493 = To Time Stamp(1:w991) -> (0:w992:timestamp)
                n494 = In Range and Coerce(upper limit=w987, x=w988, lower limit=w992) -> (In Range?=w986:bool)  [unwired: 1 out]
                n495 = case shown="False" w986 {
                  tunnel: w993 -> [w1003 w1027]
                  tunnel: [w1003 w1027] -> w976
                  frame False {
                    n496 = local read "Timeout ruedas"() -> (w1004:bool)
                    n497 = local read "Aviso no detección"() -> (w1007:string)
                    n498 = local read "Aviso temperatura"() -> (w1006:string)
                    n499 = case shown="True" w1004 {
                      selector: w1004 -> [_ w1024]
                      tunnel: ["\r" w1025] -> w1002
                      frame False {
                      }
                      frame True {
                        w1014 = "\n"
                        n500 = local read "Nº Ruedas 1"() -> (w1021:i32)
                        n501 = local read "NºRuedas 2"() -> (w1016:i32)
                        n502 = call "ErrorRuedas.vi"("Buffer Overflow"=w1024) -> ("error out"=w1026:errorcluster)
                        n503 = Number To Decimal String(number=w1021) -> (decimal integer string=w1019:string)  [unwired: 1 in]
                        n504 = Number To Decimal String(number=w1016) -> (decimal integer string=w1015:string)  [unwired: 1 in]
                        n505 = Concatenate Strings("Error Wheel sensors", "\n", "WS1 (wheels):", w1019, w1014, "WS2 (wheels):", w1015, w1014) -> (w1017:string)
                        n506 = call "Error.vi"("Error con..."=w1017, "error comunicacion 2"=w1026) -> ("String"=w1025:string)
                      }
                    }
                    n507 = local read "DC OK"() -> (w1005:string)
                    n508 = call "Cabecera.vi"() -> ("String"=w1012:string)
                    n509 = call "Adquisicion.vi"("Aviso no detección"=w1007) -> ("String"=w1011:string)
                    n510 = call "Temperatura.vi"("Aviso temperatura"=w1006) -> ("String"=w1010:string)
                    n511 = call "Fuente.vi"("DC OK"=w1005) -> ("String"=w1009:string)
                    n512 = call "FPGA.vi"("error out"=w1003) -> ("String"=w1008:string)
                    n513 = Concatenate Strings(w1012, w1011, w1010, w1009, w1008, w1002) -> (w995:string)
                    n514 = local read "Report"() -> (w994:string)
                    n515 = Get Date/Time In Seconds() -> ()  [unwired: 1 out]
                    n516 = Concatenate Strings(w995, w994) -> (w997:string)
                    n517 = local read "Max archivos"() -> (w998:u32)
                    n518 = local read "Path LOG"() -> (w1001:path)
                    n519 = local read "LOG.txt"() -> (w999:path)
                    n520 = call "Saving_LOG.vi"("Path"=w999, "Report"=w997, "Report AURA"=w995, "Path Carpeta"=w1001, "Nº Archivos Max"=w998) -> ("Report"=w1000:string)  [unwired: 9 in, 1 out]
                    n521 = local write "Report"(w1000) -> ()
                    "Ultimo TEST" <- timestamp(3608692059.513 s since 1904-01-01) ("Ultimo TEST")
                  }
                  frame True {
                  }
                }
                n522 = local read "Fallo fotocelula"() -> (w979:bool)
                n523 = Unbundle By Name(w976) -> ("status"=w977:bool)
                n524 = local read "T fuera rango"() -> (w985:bool)
                n525 = Compound Arithmetic op=OR(w977, w979) -> (w978:bool)
                n526 = local write "Reset del controlador"(w978) -> ()
                n527 = Select(t="Escape", s=w985, f="Espera") -> (s? t:f=w982:string)
                n528 = Select(t="Configuracion", s=w978, f=w982) -> (s? t:f=w980:string)
              }
            }
            n529 = call <vilib>:"Watchdog Clear.vi"("error in (no error)"=w951, "watchdogID in"=w952) -> ("error out"=w949:errorcluster)  [unwired: 5 in]
          }
          frame "Calibracion" {
            n530 = flat-sequence {
              tunnel: w1043 -> [w1227]
              tunnel: w1042 -> [w1226]
              tunnel: [w1227] -> w1041
              tunnel: [w1226] -> w1040
              frame #0 {
                n531 = local read "Report"() -> (w1223:string)
                n532 = call "Reporting_datetime.vi"() -> ("String"=w1222:string)  [unwired: 11 in]
                n533 = Concatenate Strings(w1222, "\nSTATUS: CALIBRATION\n\n\n", w1223) -> (w1225:string)
                n534 = local write "Report"(w1225) -> ()
              }
            }
            n535 = flat-sequence {
              tunnel: w1040 -> [w1047]
              tunnel: w1041 -> [w1048]
              tunnel: [w1048] -> w1036
              tunnel: [w1047] -> w1035
              tunnel: [w1045] -> w1034
              tunnel: w1036 -> [w1053]
              tunnel: w1035 -> [w1052]
              tunnel: w1034 -> [w1049]
              tunnel: [w1051] -> w1033
              tunnel: [w1050] -> w1032
              tunnel: w1033 -> [w1165]
              tunnel: w1032 -> [w1164]
              tunnel: [w1165] -> w1031
              tunnel: [w1164] -> w1030
              tunnel: [w1148] -> w1029
              tunnel: [w1147] -> w1028
              tunnel: [w1208] -> w1037
              tunnel: [w1209] -> w1038
              tunnel: w1031 -> [w1209]
              tunnel: w1030 -> [w1208]
              tunnel: w1029 -> [w1207]
              tunnel: w1028 -> [w1203]
              frame #0 {
                n536 = call "Folder_creation_calibration.vi"() -> ("path"=w1046:path, "date/time string"=w1045:string, "calibration log"=→"calibration log":path)  [unwired: 2 in]
                "Folder" <- w1046
                n537 = Create Folder(path (use dialog)=w1046) -> ()  [unwired: 2 in, 3 out]
              }
              frame #1 {
                n538 = for {
                  N: 11 -> [_]
                  shift-right: [w1078] -> w1051
                  shift-left: w1053 -> [w1077]
                  shift-right: [w1079] -> w1050
                  shift-left: w1052 -> [w1076]
                  tunnel: w1049 -> [w1055]
                  i -> [w1071]
                  n539 = xnode "Invoke Method"("FPGA VI Reference In"=w1077, "error in"=w1076) -> ("FPGA VI Reference Out"=w1075:refnum<k20>, "error out"=w1073:errorcluster)  [unwired: 1 in]
                  n540 = Increment(x=w1071) -> (x+1=w1070:i32)
                  n541 = Number To Decimal String(number=w1070) -> (decimal integer string=w1069:string)  [unwired: 1 in]
                  n542 = flat-sequence {
                    tunnel: w1075 -> [w1143]
                    tunnel: [w1143] -> w1074
                    tunnel: w1073 -> [w1142]
                    tunnel: [w1142] -> w1072
                    tunnel: w1069 -> [w1141]
                    frame #0 {
                      n543 = local read "Report"() -> (w1138:string)
                      n544 = Concatenate Strings("\nAcquiring file: ", w1141, "/11\n" ("string"), w1138) -> (w1137:string)
                      n545 = local write "Report"(w1137) -> ()
                    }
                  }
                  n546 = flat-sequence {
                    tunnel: w1072 -> [w1082]
                    tunnel: w1074 -> [w1083]
                    tunnel: [w1083] -> w1068
                    tunnel: [w1082] -> w1067
                    tunnel: [w1080] -> w1056
                    tunnel: w1055 -> [w1080]
                    tunnel: [w1097] -> w1066
                    tunnel: [w1096] -> w1065
                    tunnel: [w1095] -> w1064
                    tunnel: [w1094] -> w1063
                    tunnel: [w1093] -> w1062
                    tunnel: [w1092] -> w1061
                    tunnel: w1068 -> [w1100]
                    tunnel: w1067 -> [w1099]
                    tunnel: w1056 -> [w1084]
                    tunnel: [w1123] -> w1060
                    tunnel: [w1108] -> w1059
                    tunnel: [w1122] -> w1058
                    tunnel: [w1107] -> w1057
                    tunnel: w1066 -> [w1121]
                    tunnel: w1065 -> [w1120]
                    tunnel: w1064 -> [w1119]
                    tunnel: w1063 -> [w1118]
                    tunnel: w1062 -> [w1117]
                    tunnel: w1061 -> [w1116]
                    tunnel: w1060 -> [w1133]
                    tunnel: w1059 -> [w1132]
                    tunnel: w1058 -> [w1134]
                    tunnel: w1057 -> [w1124]
                    tunnel: [w1135] -> w1079
                    tunnel: [w1136] -> w1078
                    frame #0 {
                      n547 = Wait (ms)(milliseconds to wait=u32 1000) -> ()  [unwired: 1 out]
                    }
                    frame #1 {
                      n548 = local read "Frecuencia de muestreo y módulo CRIO"() -> (w1101:T2)
                      n549 = local read "Escaneos de la FIFO por canal"() -> (w1104:u32)
                      n550 = local read "Frecuencia de muestreo (Hz)"() -> (w1103:dbl)
                      n551 = local read "Nº de acelerómetros"() -> (w1106:i32)
                      n552 = local read "Nº inductivos"() -> (w1105:i32)
                      n553 = local read "Count(mSec)"() -> (w1102:u32)
                      n554 = Get Date/Time In Seconds() -> (seconds since 1Jan1904=→"Inicio pasada 2":timestamp)
                      n555 = Bundle("Frecuencia de muestreo y módulo CRIO"=w1101, "Count(mSec)"=w1102, "Frecuencia de muestreo (Hz)"=w1103, "Escaneos de la FIFO por canal"=w1104, "Nº inductivos"=w1105, "Nº de acelerómetros"=w1106) -> (w1098:T13)  [unwired: 1 in]
                      n556 = call "Config_calibr.vi"("error in (no error)"=w1099, "Date Folder"=w1084, "Acq parameters"=w1098, "Refnum in"=w1100) -> ("error out"=w1096:errorcluster, "Block Size"=w1094:u32, "Time to Acquire Block (ms)"=w1095:i32, "Refnum out"=w1097:refnum<k20>, "refnum out"=w1093:refnum<file>, "path"=w1086:path, "error out 2"=w1092:errorcluster)  [unwired: 1 in]
                      "path calib" <- w1086
                      n557 = Path To String(path=w1086) -> (string=w1087:string)
                      n558 = local read "Report"() -> (w1091:string)
                      n559 = Concatenate Strings("\nFile created: ", w1087, "\n", w1091) -> (w1090:string)
                      n560 = local write "Report"(w1090) -> ()
                    }
                    frame #2 {
                      n561 = local read "Inicio pasada 2"() -> (w1115:timestamp)
                      n562 = call "Acq_calibr.vi"("Refnum in"=w1121, "refnum in"=w1117, "Time to Acquire Block (ms)"=w1119, "Block Size"=w1118, "error out 3"=w1116, "error in (no error)"=w1120, "Inicio pasada 3"=w1115) -> ("refnum out 2"=w1122:refnum<file>, "Refnum out"=w1123:refnum<k20>, "Buffer Underflow 2"=w1114:bool, "error out 4"=w1108:errorcluster, "Buffer Overflow 2"=w1113:bool, "error out"=w1107:errorcluster)  [unwired: 3 in]
                      n563 = local write "Buffer Overflow"(w1113) -> ()
                      n564 = call "Reporting_error.vi"("error out 2"=w1108, "Concept"="FPGA ") -> ("Reporting"=w1110:string)  [unwired: 1 in]
                      n565 = local read "Report"() -> (w1111:string)
                      n566 = local write "Buffer Underflow"(w1114) -> ()
                      n567 = Concatenate Strings(w1110, w1111) -> (w1109:string)
                      n568 = local write "Report"(w1109) -> ()
                    }
                    frame #3 {
                      n569 = xnode "Read/Write Control"("FPGA VI Reference In"=w1133, "error in"=w1132, "Stop"=TRUE ("stop")) -> ("FPGA VI Reference Out"=w1131:refnum<k20>, "error out"=w1130:errorcluster)
                      n570 = call "Reporting_error.vi"("error out 2"=w1124, "Concept"="Saving file ") -> ("Reporting"=w1127:string)  [unwired: 1 in]
                      n571 = Close File(refnum=w1134, error in=w1124) -> ()  [unwired: 2 out]
                      n572 = local read "Report"() -> (w1126:string)
                      n573 = xnode "Invoke Method"("FPGA VI Reference In"=w1131, "error in"=w1130) -> ("FPGA VI Reference Out"=w1136:refnum<k20>, "error out"=w1135:errorcluster)
                      n574 = Concatenate Strings(w1127, w1126) -> (w1128:string)
                      n575 = local write "Report"(w1128) -> ()
                    }
                  }
                }
              }
              frame #2 {
                n576 = local read "Frecuencia de muestreo (Hz)"() -> (w1160:dbl)
                n577 = local read "Nº de acelerómetros"() -> (w1151:i32)
                n578 = local read "Nº inductivos"() -> (w1150:i32)
                n579 = local read "Pattern amplitude (g)"() -> (w1152:dbl)
                n580 = local read "Pattern frequency (Hz)"() -> (w1153:dbl)
                n581 = local read "Folder"() -> (w1163:path)
                n582 = Add(x=w1151, y=w1150) -> (x+y=w1149:i32)
                n583 = call <vilib>:"Recursive File List.vi"("Folder Path"=w1163) -> ("All Files in Dir"=w1162:path[])  [unwired: 6 in, 4 out]
                n584 = local read "Report"() -> (w1145:string)
                n585 = call "Acel_calib_detector.vi"("Frecuencia\nmuestreo"=w1160, "Pattern frequency (Hz)"=w1153, "Nº canales"=w1149, "All Files in Dir"=w1162) -> ("Continue calibrating?"=w1144:bool, "Reporting"=w1159:string, "Acceler.\ndetected"=w1148:i32, "Acel Cal measurements"=w1161:sgl[][])
                n586 = Concatenate Strings(w1159, w1145) -> (w1146:string)
                n587 = local write "Report"(w1146) -> ()
                n588 = case shown="True" w1144 {
                  tunnel: w1161 -> [_ w1179]
                  tunnel: w1160 -> [_ w1177]
                  tunnel: [w1166 w1176] -> w1156
                  tunnel: [w1166 w1175] -> w1155
                  tunnel: [w1166 w1174] -> w1154
                  tunnel: w1153 -> [_ w1173]
                  tunnel: w1152 -> [_ w1172]
                  tunnel: [-1.0 ("Calibration parameter") w1171] -> w1147
                  frame False {
                    w1166 = "" ("Reporting2")
                  }
                  frame True {
                    n589 = local read "Report"() -> (w1169:string)
                    n590 = call "Acel_calib_frequency.vi"("Pattern frequency (Hz)"=w1173, "Frecuencia\nmuestreo"=w1177, "Acel Cal measurements in"=w1179) -> ("Valid frequency"=w1168:bool, "Reporting2"=w1176:string, "Acel Cal measurements out"=w1178:sgl[][])  [unwired: 1 in, 1 out]
                    n591 = Concatenate Strings(w1176, w1169) -> (w1170:string)
                    n592 = local write "Report"(w1170) -> ()
                    n593 = case shown="True" w1168 {
                      tunnel: w1178 -> [_ w1192]
                      tunnel: w1177 -> [_ w1191]
                      tunnel: [w1180 w1189] -> w1175
                      tunnel: [w1180 w1188] -> w1174
                      tunnel: w1173 -> [_ w1187]
                      tunnel: w1172 -> [_ w1186]
                      tunnel: [-1.0 ("Calibration parameter") w1185] -> w1171
                      frame False {
                        w1180 = "" ("Reporting 3")
                      }
                      frame True {
                        n594 = call "Acel_calib_noise_files_out.vi"("Pattern frequency (Hz)"=w1187, "Frecuencia\nmuestreo"=w1191, "Acel Cal measurements in"=w1192) -> ("Measurements OK"=w1182:bool, "Reporting 3"=w1189:string, "Acel Cal measurements out 2"=w1190:sgl[][])  [unwired: 6 in]
                        n595 = local read "Report"() -> (w1184:string)
                        n596 = Concatenate Strings(w1189, w1184) -> (w1183:string)
                        n597 = local write "Report"(w1183) -> ()
                        n598 = case shown="True" w1182 {
                          tunnel: w1191 -> [_ w1202]
                          tunnel: w1190 -> [_ w1201]
                          tunnel: ["" ("Reporting 4") w1200] -> w1188
                          tunnel: w1187 -> [_ w1199]
                          tunnel: w1186 -> [_ w1198]
                          tunnel: [-1.0 ("Calibration parameter") w1197] -> w1185
                          frame False {
                          }
                          frame True {
                            n599 = call "Acel_calib_calib.vi"("Acel Cal measurements in"=w1201, "Frecuencia\nmuestreo"=w1202, "Pattern frequency (Hz)"=w1199, "Pattern\namplitude"=w1198) -> ("Calibration parameter"=w1197:dbl, "Reporting 4"=w1200:string)  [unwired: 7 in, 3 out]
                            n600 = local read "Report"() -> (w1195:string)
                            n601 = Concatenate Strings(w1200, w1195) -> (w1196:string)
                            n602 = local write "Report"(w1196) -> ()
                          }
                        }
                      }
                    }
                  }
                }
                n603 = local read "calibration log"() -> (w1157:path)
                n604 = Concatenate Strings(w1159, w1156, w1155, w1154) -> (w1158:string)
                n605 = Write to Text File(file (use dialog)=w1157, text=w1158) -> ()  [unwired: 2 in, 3 out]
              }
              frame #3 {
                n606 = local read "Save calibration"() -> (w1204:bool)
                n607 = Add(x=w1207, y=8) -> (x+y=w1205:i32)
                n608 = case shown="True" w1204 {
                  tunnel: w1205 -> [_ w1219]
                  tunnel: w1203 -> [_ w1212]
                  frame False {
                  }
                  frame True {
                    w1220 = "Parametros"  # Key 1
                    n609 = local read "configuration file path"() -> (w1213:path)
                    n610 = Number To Decimal String(number=w1219) -> (decimal integer string=w1221:string)  [unwired: 1 in]
                    n611 = Concatenate Strings(w1220, w1221) -> (w1211:string)
                    n612 = call <vilib>:"Open Config Data.vi"("create file if necessary (T)"=TRUE, "configuration file path"=w1213) -> ("error out"=w1214:errorcluster, "refnum"=w1215:T14)  [unwired: 1 in, 7 out]
                    n613 = call-poly <vilib>:"Write Key.vi"("section"="Adquisicion", "error in (no error)"=w1214, "value"=w1212, "key"=w1211, "refnum"=w1215) -> ("error out"=w1218:errorcluster, "refnum out"=w1217:T14)  [unwired: 3 in, 2 out]
                    n614 = call <vilib>:"Close Config Data.vi"("error in (no error)"=w1218, "refnum"=w1217) -> ()  [unwired: 8 in, 2 out]
                  }
                }
              }
            }
          }
          frame "UPS" {
            n615 = node-c288() -> (w1234:T7)  [unwired: 4 in]
            n616 = timed-loop {
              timing: w1234 -> [_]
              timing-out: [_] -> w1233
              tunnel: w1232 -> [w1239]
              tunnel: w1231 -> [w1238]
              tunnel: [w1237] -> w1229
              tunnel: [w1236] -> w1228
              stop <- w1235 stop-if-true
              n617 = node-c288() -> ()  [unwired: 1 in, 1 out]
              n618 = xnode "Read/Write Control"("FPGA VI Reference In"=w1239, "error in"=w1238) -> ("FPGA VI Reference Out"=w1237:refnum<k20>, "error out"=w1236:errorcluster, "DC OK"=w1235:bool)
              n619 = node-c288() -> ()  [unwired: 1 in, 1 out]
            }
            n620 = node-c288(w1233) -> ()  [unwired: 1 out]
          }
        }
        "error manipulacion archivos" <- w96
        n621 = local read "Parar la aplicación"() -> (w94:bool)
      }
      n622 = xnode "Close FPGA VI Reference"("FPGA VI Reference In"=w86, "error in"=w85) -> ("error out"=→"error FPGA":errorcluster)
    }
    frame #3 {
      n623 = local read "RFID_ID"() -> (w1246:refnum<k5>)
      n624 = call "LH6HD.vi"("Action"=enum16{"Init", "Start", "Read", "Stop", "Exit"}."Stop") -> ("error out"=→"RFID_LR6_Error":errorcluster)  [unwired: 9 in, 1 out]
      n625 = TCP Close Connection(connection ID=w1246) -> (error out=→"RFID_Error":errorcluster)  [unwired: 1 in, 2 out]
    }
  }
